vi "Strain Measurement.vi"(0 "Function":T5=enum."Update Sequence Status", 1 "Stress Sequence Parameters":T6={"Max Motor Position"=1380.0, "# Intermediate Points"=5000, "Initial Direction"=enum."Tension"} caption="Stress Parameters" {"# Intermediate Points" max=1390}, 2 "Which Program?":T1, 5 "Notifiers":T9, 7 "Message Queues":T22, 9 "Refnums":T7, 11 "error in (no error)":errorcluster, 12 "Track":bool) -> (6 "Sequence Progress":cluster{i32[], "Y":dbl[]}[](graph)=[{[0, 1, 2], "Y"=[-3.816391647148976e-15, -49.99999999999999, 0.0]}, {[3], "Y"=[50.0]}, {[4], "Y"=[-3.816391647148976e-15]}] caption="Strain Measurement Status", 15 "error out":errorcluster)   [LabVIEW 2014]
uses:
  support/Message Queue/All Message Queues.ctl
  support/Message Queue/Message Cluster.ctl
  support/Notifiers/Notifiers.ctl
  support/Message Handler Loop Notifiers.ctl
  Hardware Control/Parameter Analyzer/Parameter Analyzer Notifiers.ctl
  Hardware Control/Switching Matrix/Switching Matrix Notifiers.ctl
  Hardware Control/Stress Control/StressControl Notifiers.ctl
  Hardware Control/Spectrometer/Spectrometer Notifiers.ctl
  Hardware Control/Switches and Mirrors/SwitchesMirrors Notifiers.ctl
  Hardware Control/Camera/Camera Notifiers.ctl
  Hardware Control/XYZ Stage/XYZ Notifications.ctl
  Hardware Control/Autofocus/Autofocus Notifiers.ctl
  Optoelectronic Measurement/Optoelectronic Notifiers.ctl
  Save Data/SaveData Notifiers.ctl
  Instrument Sequence/Instrument Sequence Notifiers.ctl
  Strain Measurement Refnums.ctl
  Instrument Sequence/Action.ctl
  Instrument Sequence/Instrument List.ctl
  Plot Data/Electrical Data Plot Refnums.ctl
  Strain Measurement Function.ctl
  Instrument Sequence/Instrument Steps.ctl
  Instrument Sequence/Instrument Stequence - Which Program.ctl
  Hardware Control/Autofocus/AutoFocus Data.ctl
  Hardware Control/Autofocus/AutoFocus Config.ctl
  Hardware Control/Autofocus/ZScan.ctl
  <vilib>/Analysis/Matrix/Datatypes/RealMatrix.ctl
  Hardware Control/Autofocus/AutoFocus Refnums.ctl
  Hardware Control/Autofocus/Target Refnums.ctl
  Hardware Control/Autofocus/AutoFocus Initialize.ctl
  Hardware Control/Switches and Mirrors/SwitchesMirrors Config.ctl
  Hardware Control/Switches and Mirrors/SwitchesMirrors Status.ctl
  support/Message Queue/Message Queue.lvlib
  <vilib>/Analysis/Matrix/NI_Matrix.lvlib
panel:
  in  "Strain Measurement - Pause":bool
  out "Device ID":string caption="Instrument Sequence - Device ID"
  out "Device Information":string
  out "Instrument Steps":T2
  # "LICENSED MATERIALS – PROPERTY OF IBM\nCopyright IBM Corp. 2016,\nALL RIGHTS RESERVED"
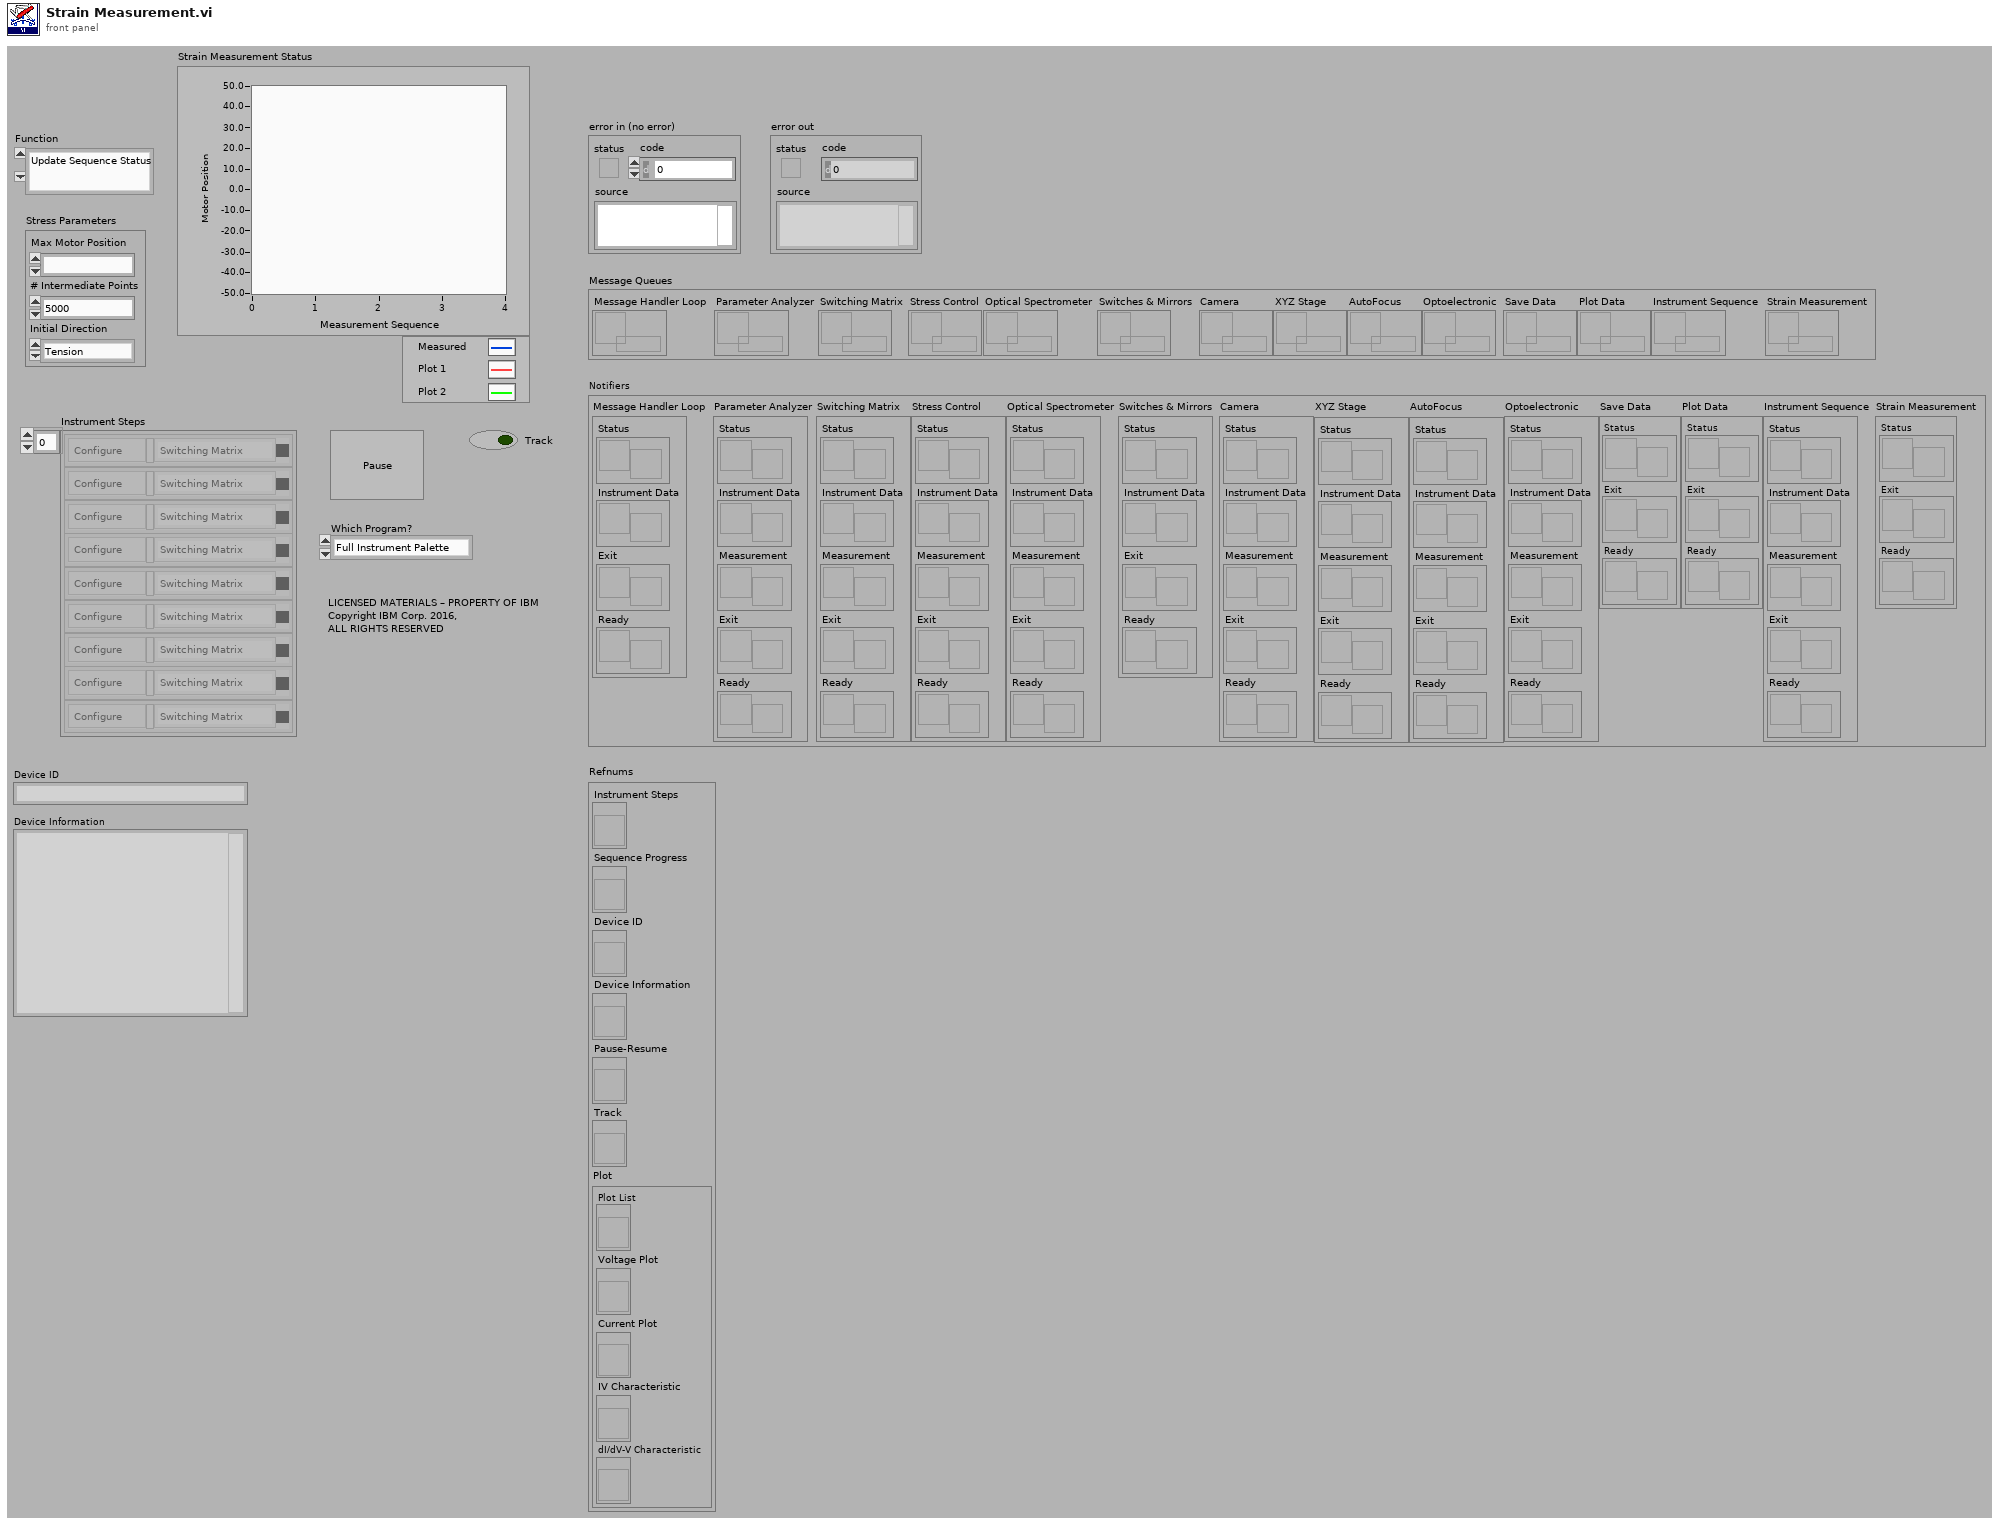
[diagram p1: front panel]
types:
  T1 = typedef "Instrument Stequence - Which Program.ctl" = enum16{"Full Instrument Palette", "Strain Electrical"}
  T2 = typedef "Instrument Steps.ctl" = cluster{"Action":T3, "Configuration":variant, "Instrument":T4, "Status":enum8{"False", "True", "Mixed"}}[]
  T3 = typedef "Action.ctl" = enum32{"Configure", "Measure"}
  T4 = typedef "Instrument List.ctl" = enum32{"Unknown Instrument", "Switching Matrix", "Parameter Analyzer", "Optical Spectrometer", "Optoelectronic", "Autofocus"}
  T5 = typedef "Strain Measurement Function.ctl" = enum16{"Get Stress Controller Status", "Define Strain Sequence", "Update Track", "Decide on Track", "Reset Strain Sequence", "Start Strain Measurement", "Set Strain Sequence Step", "Add Instrument Sequence Step", "Delete Instrument Sequence Step", "Clear Instrument Sequence", "Reset Instrument Sequence", "Load Instrument Sequence", "Save Instrument Sequence", "Measure Instrument Sequence", "Choose What Next", "Configure Stress Control", "Set Workspace Data", "Save to Workspace", "Update Sequence Status", "Pause", "Stop", "Update Refnums"}
  T6 = cluster{"Max Motor Position":ext, "# Intermediate Points":u32, "Initial Direction":enum16{"Tension", "Compression"}}
  T7 = typedef "Strain Measurement Refnums.ctl" = cluster{"Instrument Steps":refnum<vi>, "Sequence Progress":refnum<vi>, "Device ID":refnum<vi>, "Device Information":refnum<vi>, "Pause-Resume":refnum<vi>, "Track":refnum<vi>, "Plot":T8}
  T8 = typedef "Electrical Data Plot Refnums.ctl" = cluster{"Plot List":refnum<vi>, "Voltage Plot":refnum<vi>, "Current Plot":refnum<vi>, "IV Characteristic":refnum<vi>, "dI/dV-V Characteristic":refnum<vi>}
  T9 = typedef "Notifiers.ctl" = cluster{"Message Handler Loop":T10, "Parameter Analyzer":T11, "Switching Matrix":T12, "Stress Control":T13, "Optical Spectrometer":T14, "Switches & Mirrors":T15, "Camera":T16, "XYZ Stage":T17, "AutoFocus":T18, "Optoelectronic":T19, "Save Data":T20, "Plot Data":T20, "Instrument Sequence":T21, "Strain Measurement":cluster{"Status":refnum<notifier>, "Exit":refnum<notifier>, "Ready":refnum<notifier>}}
  T10 = typedef "Message Handler Loop Notifiers.ctl" = cluster{"Status":refnum<notifier>, "Instrument Data":refnum<notifier>, "Exit":refnum<notifier>, "Ready":refnum<notifier>}
  T11 = typedef "Parameter Analyzer Notifiers.ctl" = cluster{"Status":refnum<notifier>, "Instrument Data":refnum<notifier>, "Measurement":refnum<notifier>, "Exit":refnum<notifier>, "Ready":refnum<notifier>}
  T12 = typedef "Switching Matrix Notifiers.ctl" = cluster{"Status":refnum<notifier>, "Instrument Data":refnum<notifier>, "Measurement":refnum<notifier>, "Exit":refnum<notifier>, "Ready":refnum<notifier>}
  T13 = typedef "StressControl Notifiers.ctl" = cluster{"Status":refnum<notifier>, "Instrument Data":refnum<notifier>, "Measurement":refnum<notifier>, "Exit":refnum<notifier>, "Ready":refnum<notifier>}
  T14 = typedef "Spectrometer Notifiers.ctl" = cluster{"Status":refnum<notifier>, "Instrument Data":refnum<notifier>, "Measurement":refnum<notifier>, "Exit":refnum<notifier>, "Ready":refnum<notifier>}
  T15 = typedef "SwitchesMirrors Notifiers.ctl" = cluster{"Status":refnum<notifier>, "Instrument Data":refnum<notifier>, "Exit":refnum<notifier>, "Ready":refnum<notifier>}
  T16 = typedef "Camera Notifiers.ctl" = cluster{"Status":refnum<notifier>, "Instrument Data":refnum<notifier>, "Measurement":refnum<notifier>, "Exit":refnum<notifier>, "Ready":refnum<notifier>}
  T17 = typedef "XYZ Notifications.ctl" = cluster{"Status":refnum<notifier>, "Instrument Data":refnum<notifier>, "Measurement":refnum<notifier>, "Exit":refnum<notifier>, "Ready":refnum<notifier>}
  T18 = typedef "Autofocus Notifiers.ctl" = cluster{"Status":refnum<notifier>, "Instrument Data":refnum<notifier>, "Measurement":refnum<notifier>, "Exit":refnum<notifier>, "Ready":refnum<notifier>}
  T19 = typedef "Optoelectronic Notifiers.ctl" = cluster{"Status":refnum<notifier>, "Instrument Data":refnum<notifier>, "Measurement":refnum<notifier>, "Exit":refnum<notifier>, "Ready":refnum<notifier>}
  T20 = typedef "SaveData Notifiers.ctl" = cluster{"Status":refnum<notifier>, "Exit":refnum<notifier>, "Ready":refnum<notifier>}
  T21 = typedef "Instrument Sequence Notifiers.ctl" = cluster{"Status":refnum<notifier>, "Instrument Data":refnum<notifier>, "Measurement":refnum<notifier>, "Exit":refnum<notifier>, "Ready":refnum<notifier>}
  T22 = typedef "Message Queue.lvlib/All Message Queues.ctl" = cluster{"Message Handler Loop":refnum<queue>, "Parameter Analyzer":refnum<queue>, "Switching Matrix":refnum<queue>, "Stress Control":refnum<queue>, "Optical Spectrometer":refnum<queue>, "Switches & Mirrors":refnum<queue>, "Camera":refnum<queue>, "XYZ Stage":refnum<queue>, "AutoFocus":refnum<queue>, "Optoelectronic":refnum<queue>, "Save Data":refnum<queue>, "Plot Data":refnum<queue>, "Instrument Sequence":refnum<queue>, "Strain Measurement":refnum<queue>}
  T23 = cluster{"Wanna Track?":bool, "Makes Sense?":bool}
  T24 = typedef "AutoFocus Data.ctl" = cluster{"Configuration":T25, "Refnums":T28, "Initialize":T30}
  T25 = typedef "AutoFocus Config.ctl" = cluster{"Matching Criteria":cluster{"Minimum Score":sgl, "Color Score Weight":sgl, "Minimum Contrast":i32, "Match Mode":u32, "Match Feature Mode":u32, "Subpixel Accuracy":bool, "Color Sensitivity":u32, "Search Strategy":u32}, "Z Scan Parameters":T26, "Displacement":dbl, "Transformation Matrix":T27}
  T26 = typedef "ZScan.ctl" = cluster{"Z Range":ext, "Resolution":dbl, "Initial Direction":enum16{"Up", "Down"}, "Focus Threshold":dbl, "Ascent Constant":dbl}
  T27 = typedef "NI_Matrix.lvlib/RealMatrix.ctl" = dbl[][]
  T28 = typedef "AutoFocus Refnums.ctl" = cluster{"Instrument Status":refnum<vi>, "Matching Criteria":refnum<vi>, "Z Scan Parameters":refnum<vi>, "Distance":refnum<vi>, "Transformation Matrix":refnum<vi>, "Match and Edge":T29, "Matching Curves":refnum<vi>, "Tracking":refnum<vi>, "Focus":refnum<vi>, "Find Focus":refnum<vi>, "Set Target":refnum<vi>, "Link Stage & Camera":refnum<vi>, "Align":refnum<vi>}
  T29 = typedef "Target Refnums.ctl" = cluster{"Image":refnum<vi>, "Target":refnum<vi>, "Edge":refnum<vi>, "Target Data":refnum<vi>}
  T30 = typedef "AutoFocus Initialize.ctl" = cluster{"Update Refnums":bool, "Allocate Image Memory":bool, "Set Match Criteria":bool, "Link Stage & Camera":bool, "Set Target":bool, "Find Target":bool}
  T31 = enum8{"Enabled", "Disabled", "Disabled and Grayed Out"}
  T32 = typedef "SwitchesMirrors Config.ctl" = cluster{"Relay VISA Session":refnum<visa-resource-name>, "Switches":T33, "Delays (ms)":cluster{"Laser":u32, "Video":u32}}
  T33 = typedef "SwitchesMirrors Status.ctl" = cluster{"Laser":bool, "Video":bool}
  T34 = typedef "StressControl Config.ctl" = cluster{"Stress Control VISA Session":refnum<visa-resource-name>, "Axis":i32, "Motion":u16, "Destination (°)":dbl, "Speed (°/s)":dbl, "Position (°)":dbl}
  T35 = typedef "SaveData Workspace Info.ctl" = cluster{"Device Name":string, "Device Info":string, "Path":path}
  T36 = typedef "StressControl Data.ctl" = cluster{"Configuration":T34, "Refnums":T37, "Initialization":T38}
  T37 = typedef "StressControl Refnums.ctl" = cluster{"Instrument Status":refnum<vi>, "Position":refnum<vi>, "Mecahnism Motion":refnum<vi>, "Destination":refnum<vi>, "Apply Stress":refnum<vi>, "Stop":refnum<vi>, "Stress Control VISA":refnum<vi>}
  T38 = typedef "StressControl Initialization.ctl" = cluster{"Update Visa Session":bool, "Update Configuration":bool, "Update Refnums":bool, "Get Position":bool}
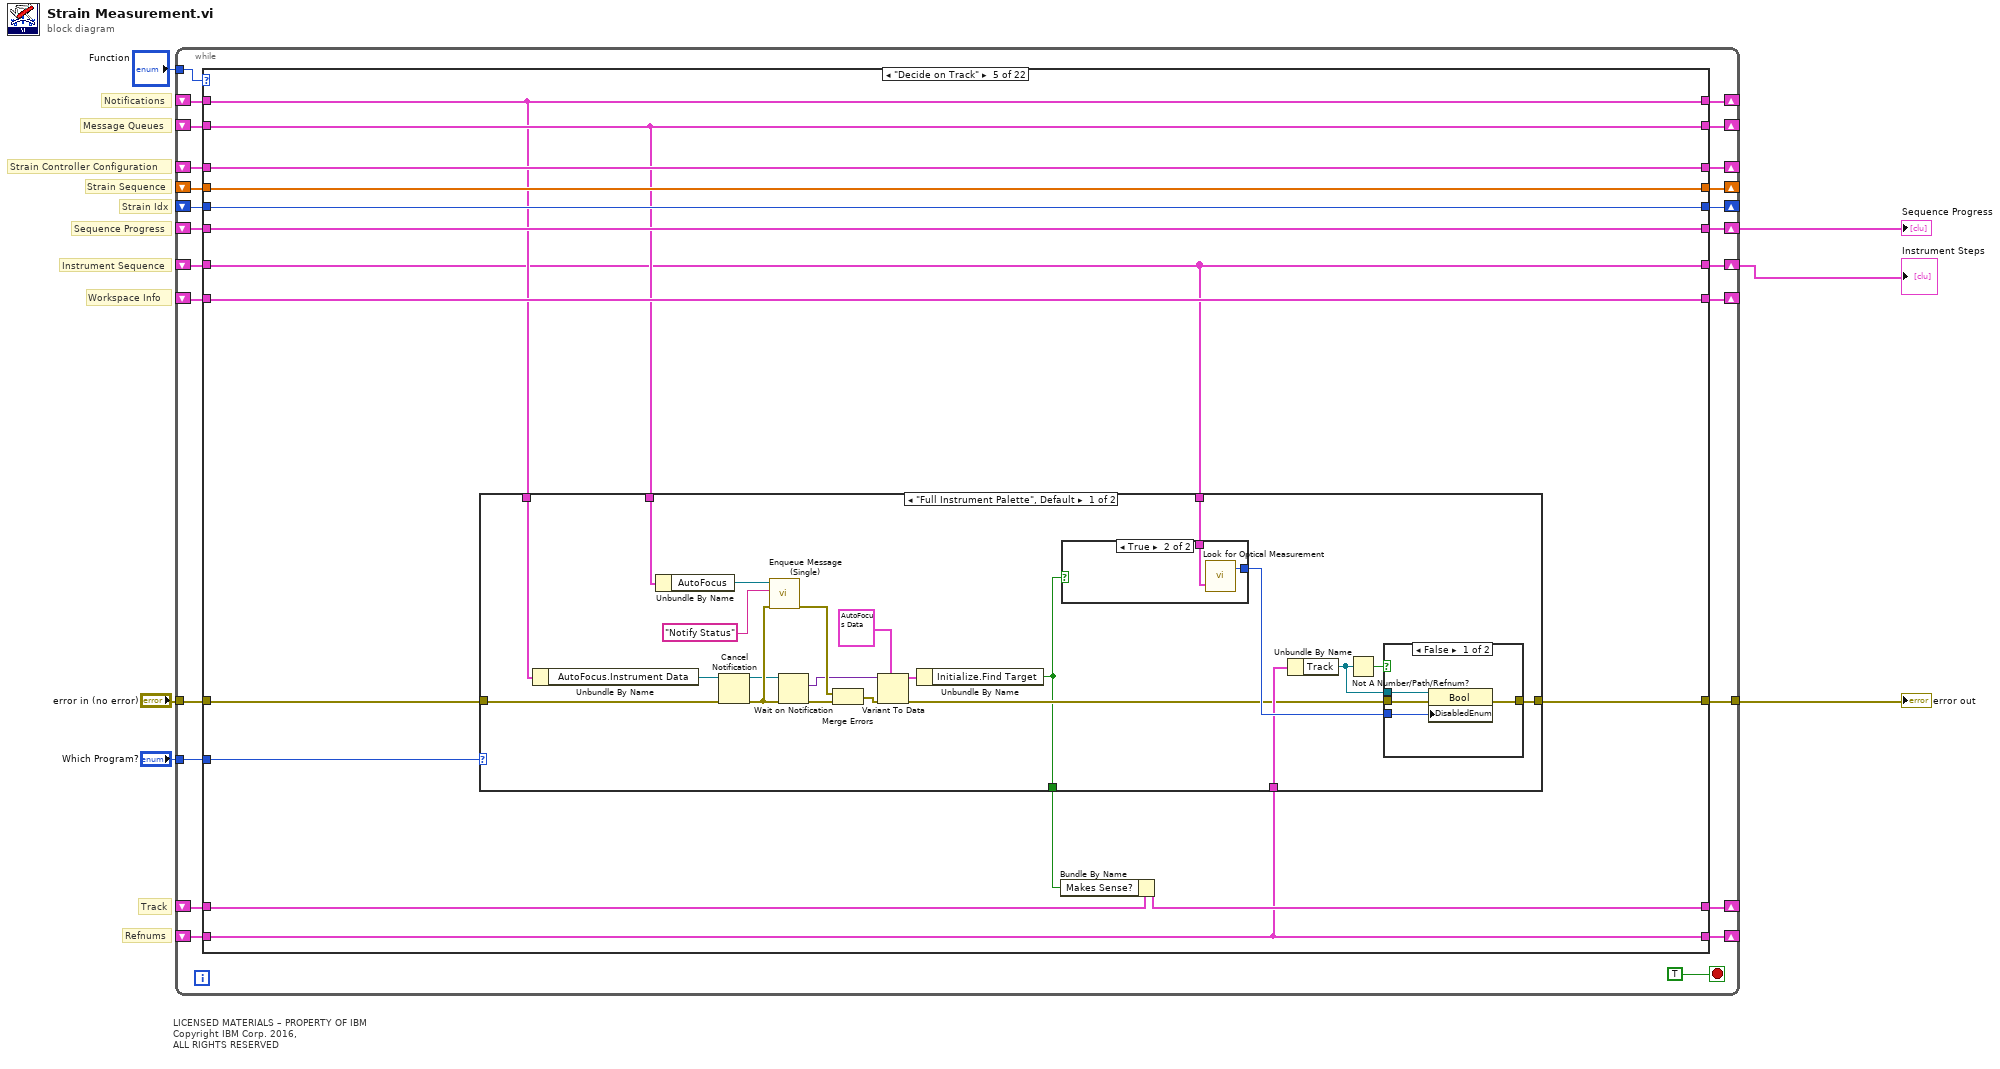
[diagram p0: block diagram]
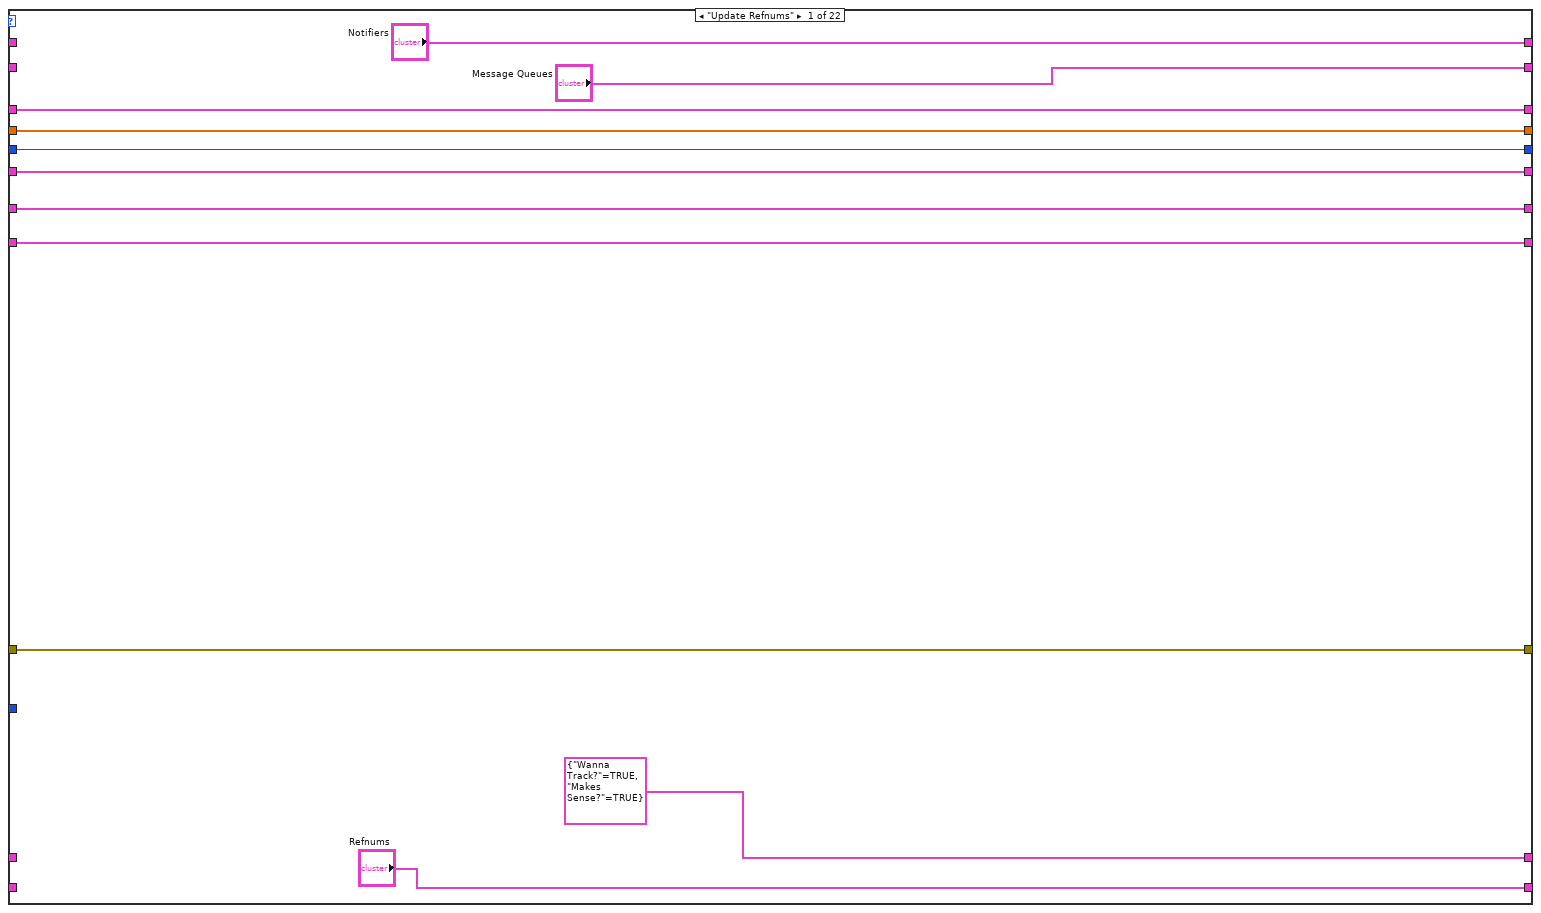
[diagram p2: hidden frame]
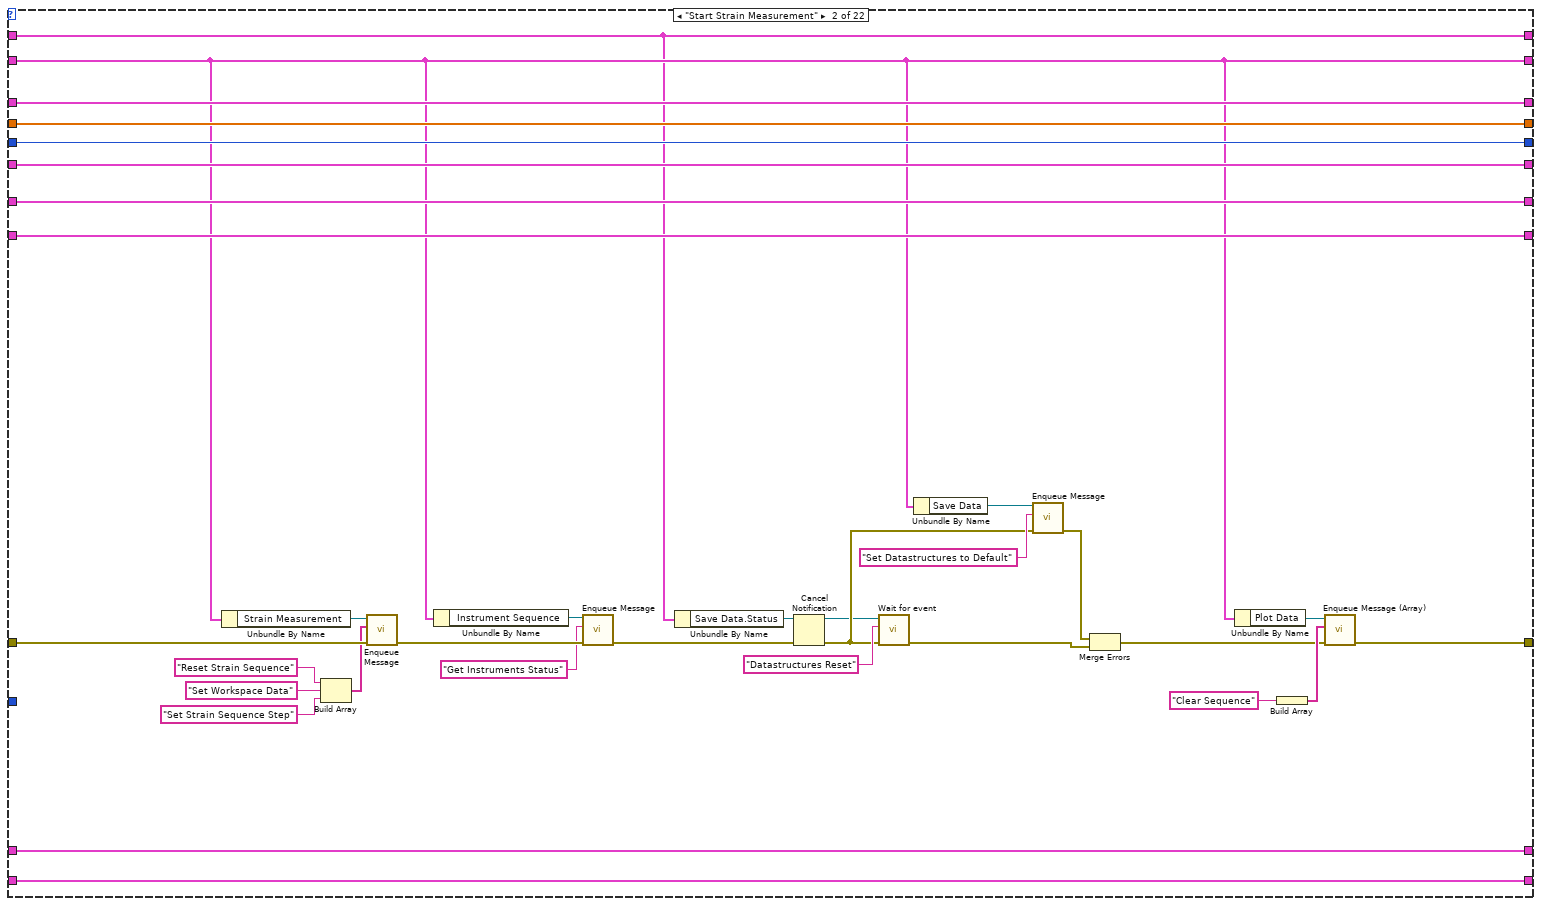
[diagram p3: hidden frame]
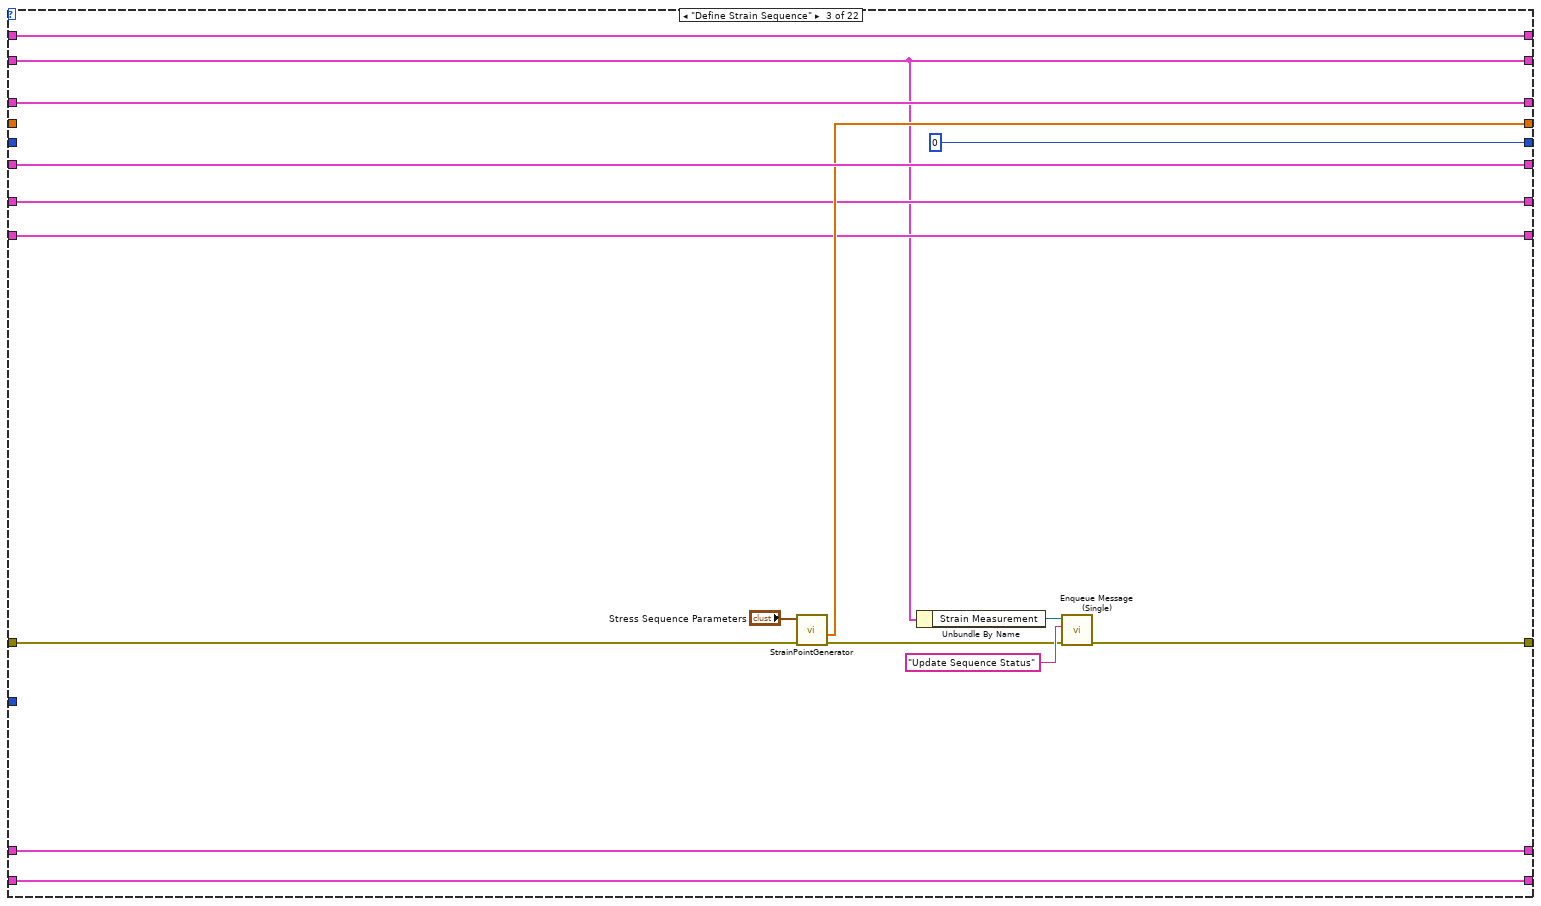
[diagram p4: hidden frame]
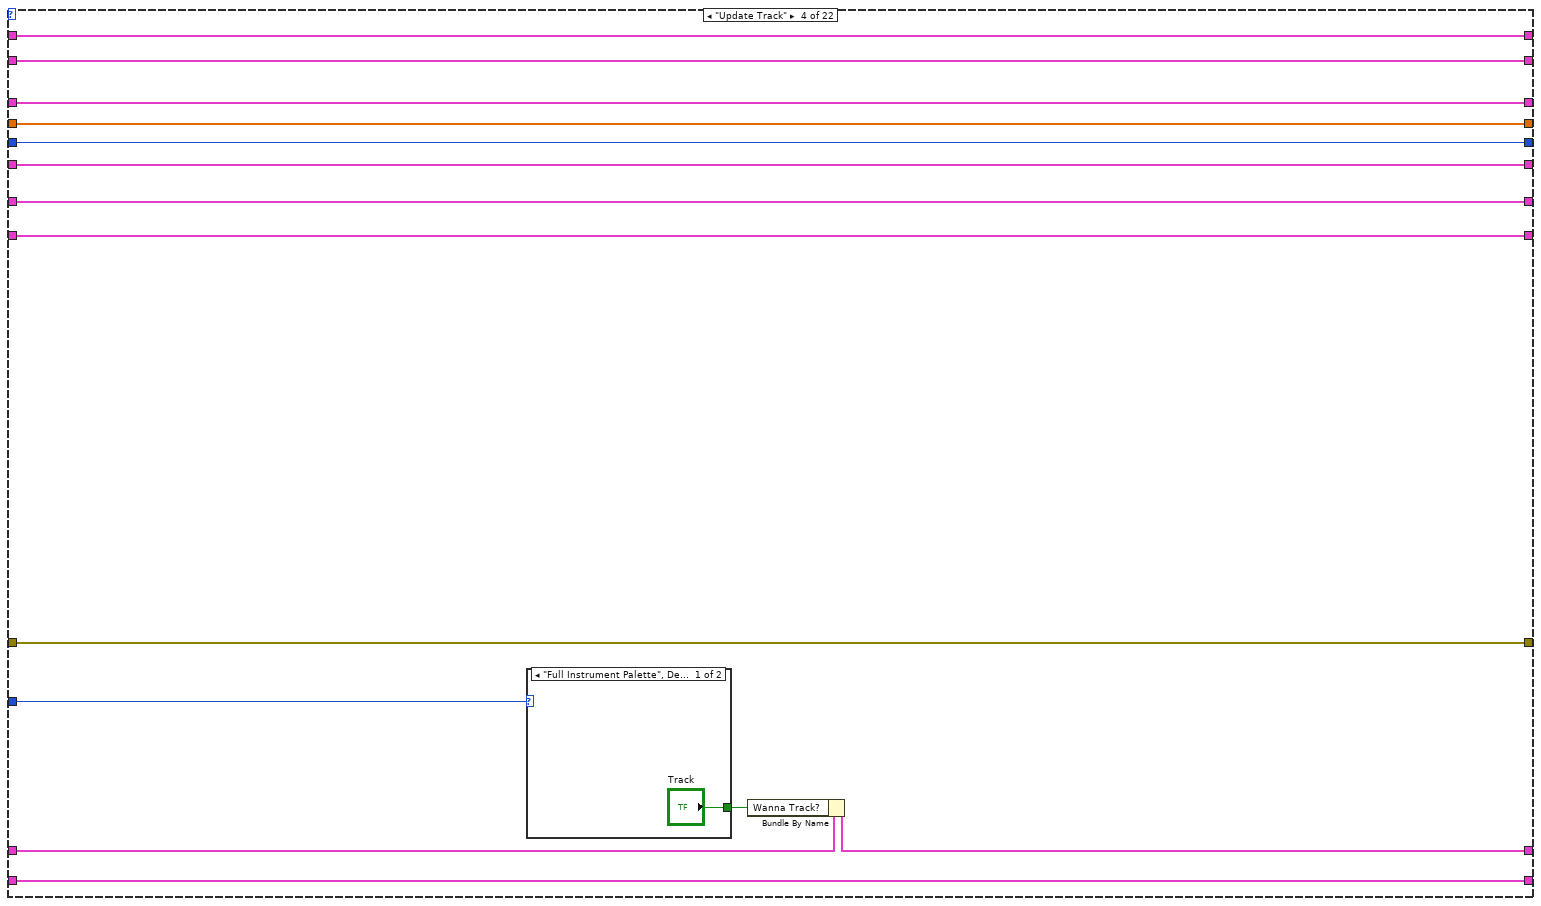
[diagram p5: hidden frame]
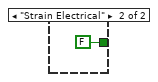
[diagram p6: hidden frame]
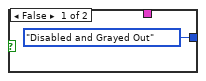
[diagram p7: hidden frame]
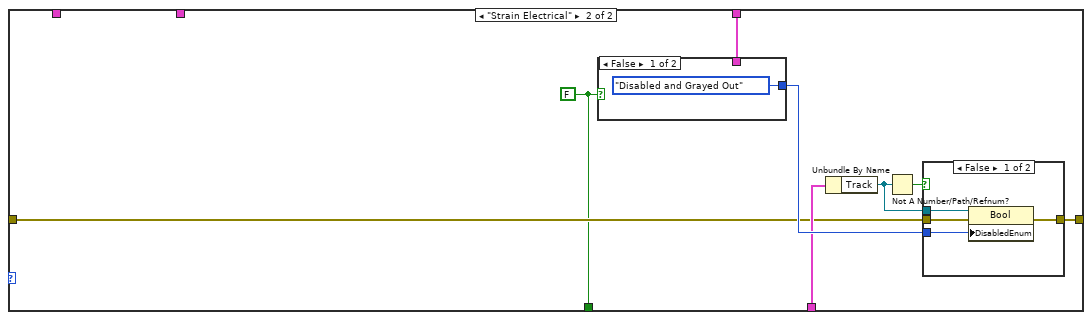
[diagram p9: hidden frame]
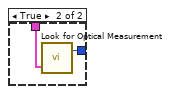
[diagram p10: hidden frame]
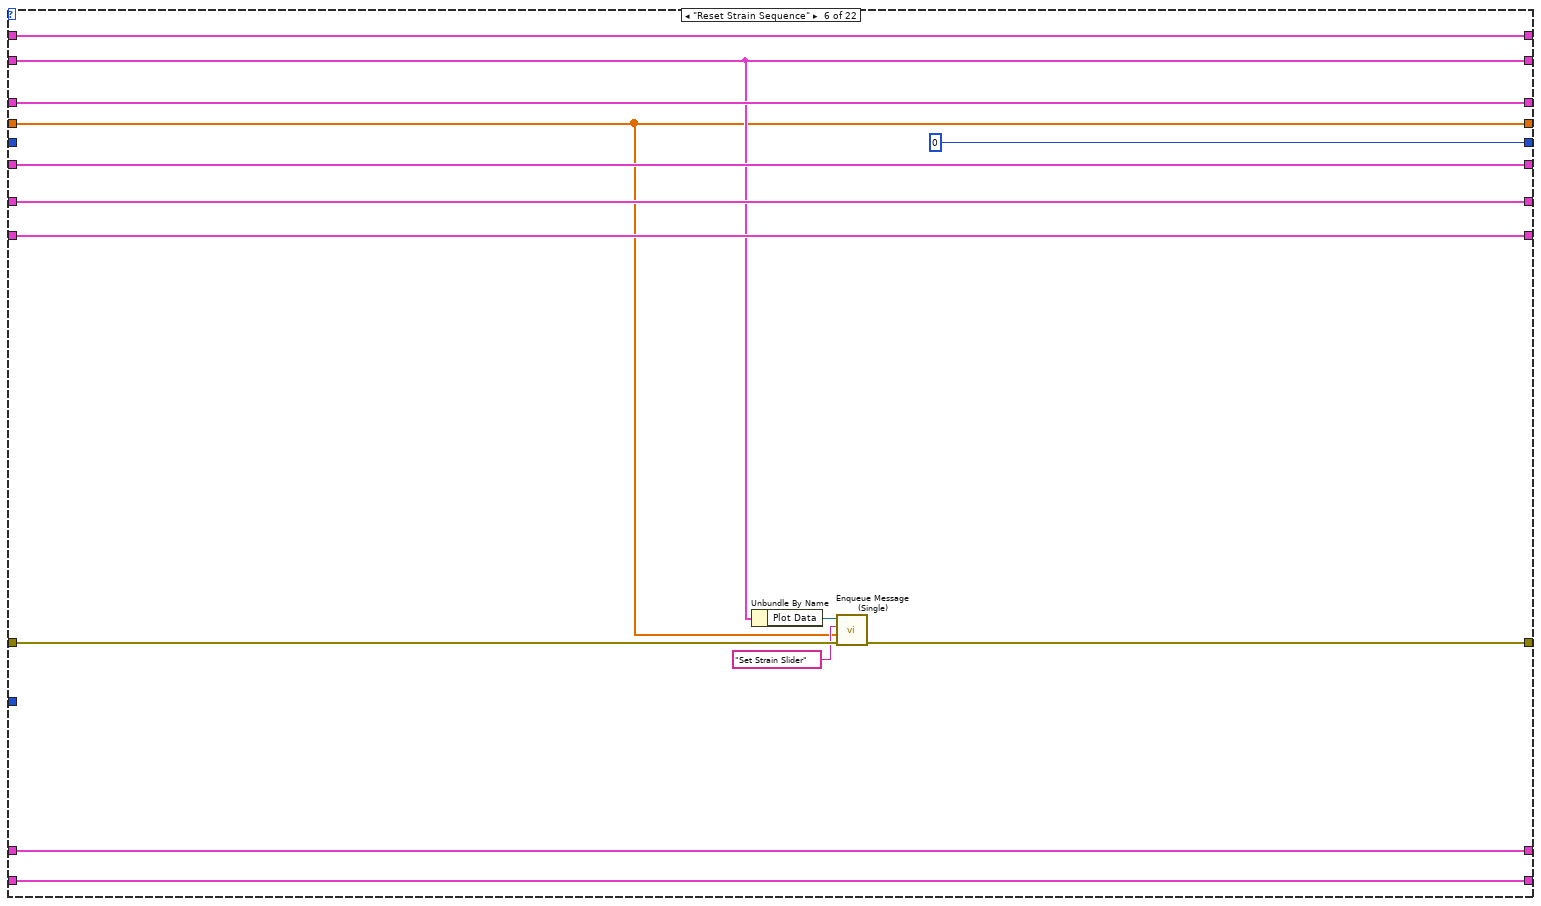
[diagram p12: hidden frame]
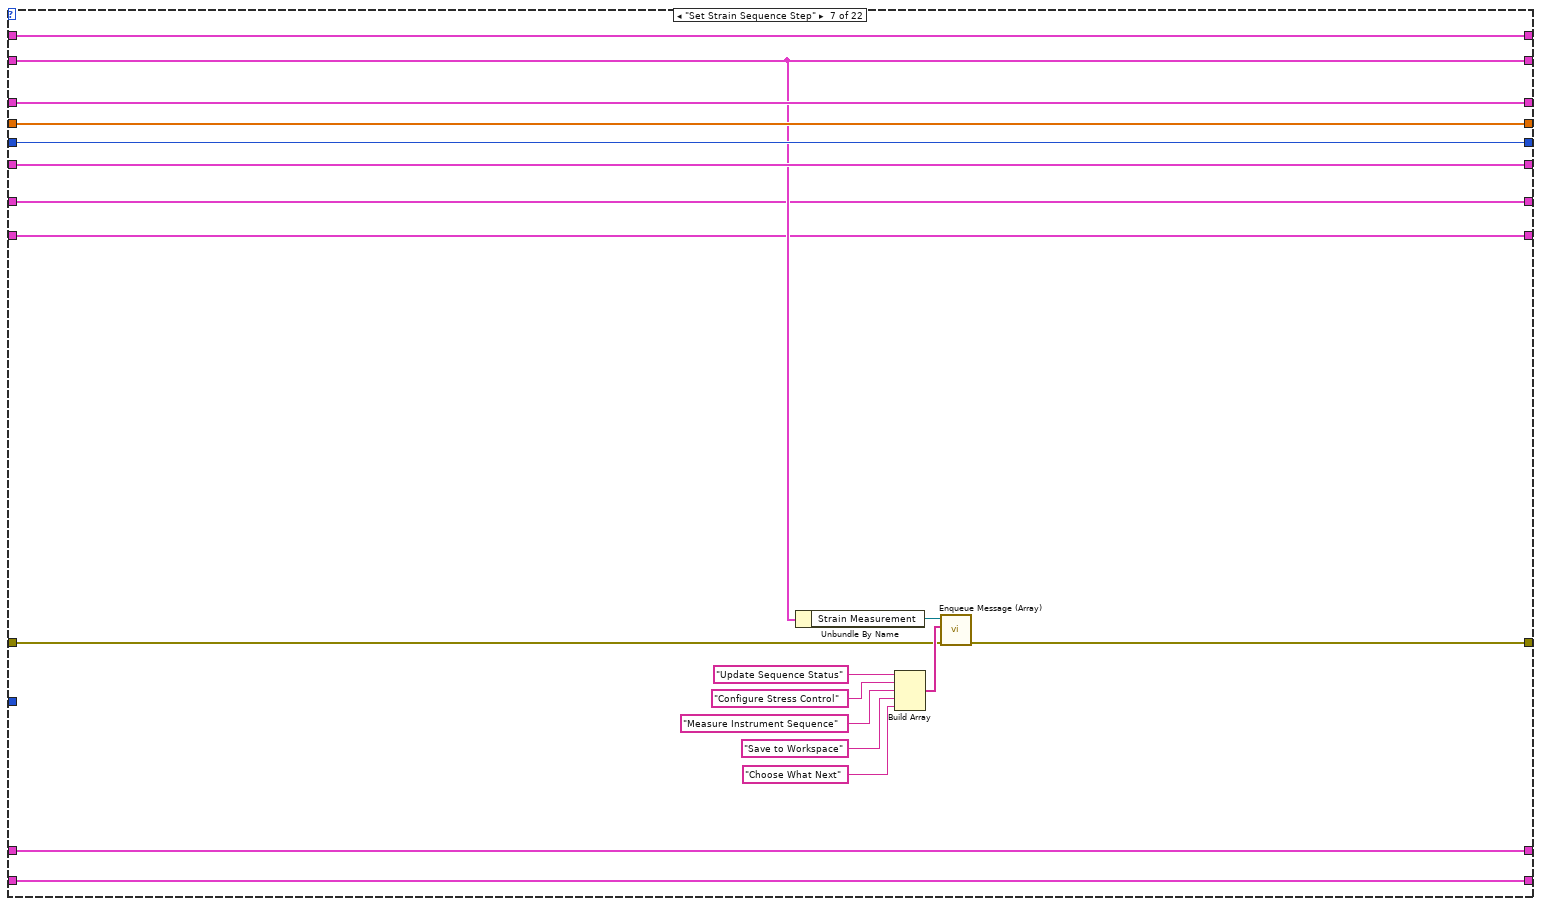
[diagram p13: hidden frame]
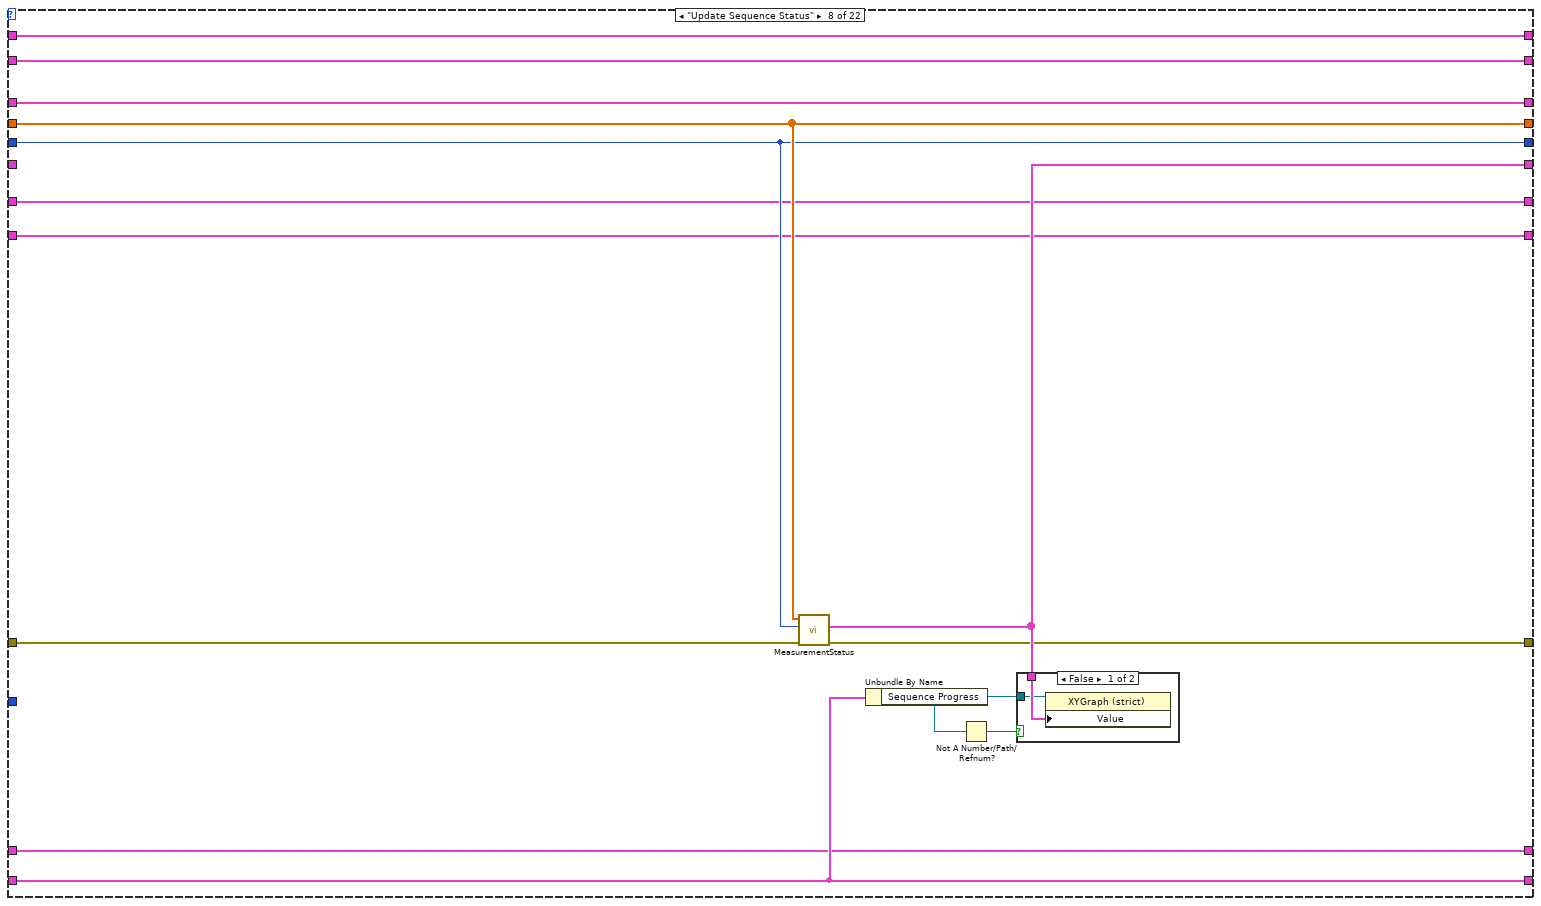
[diagram p14: hidden frame]
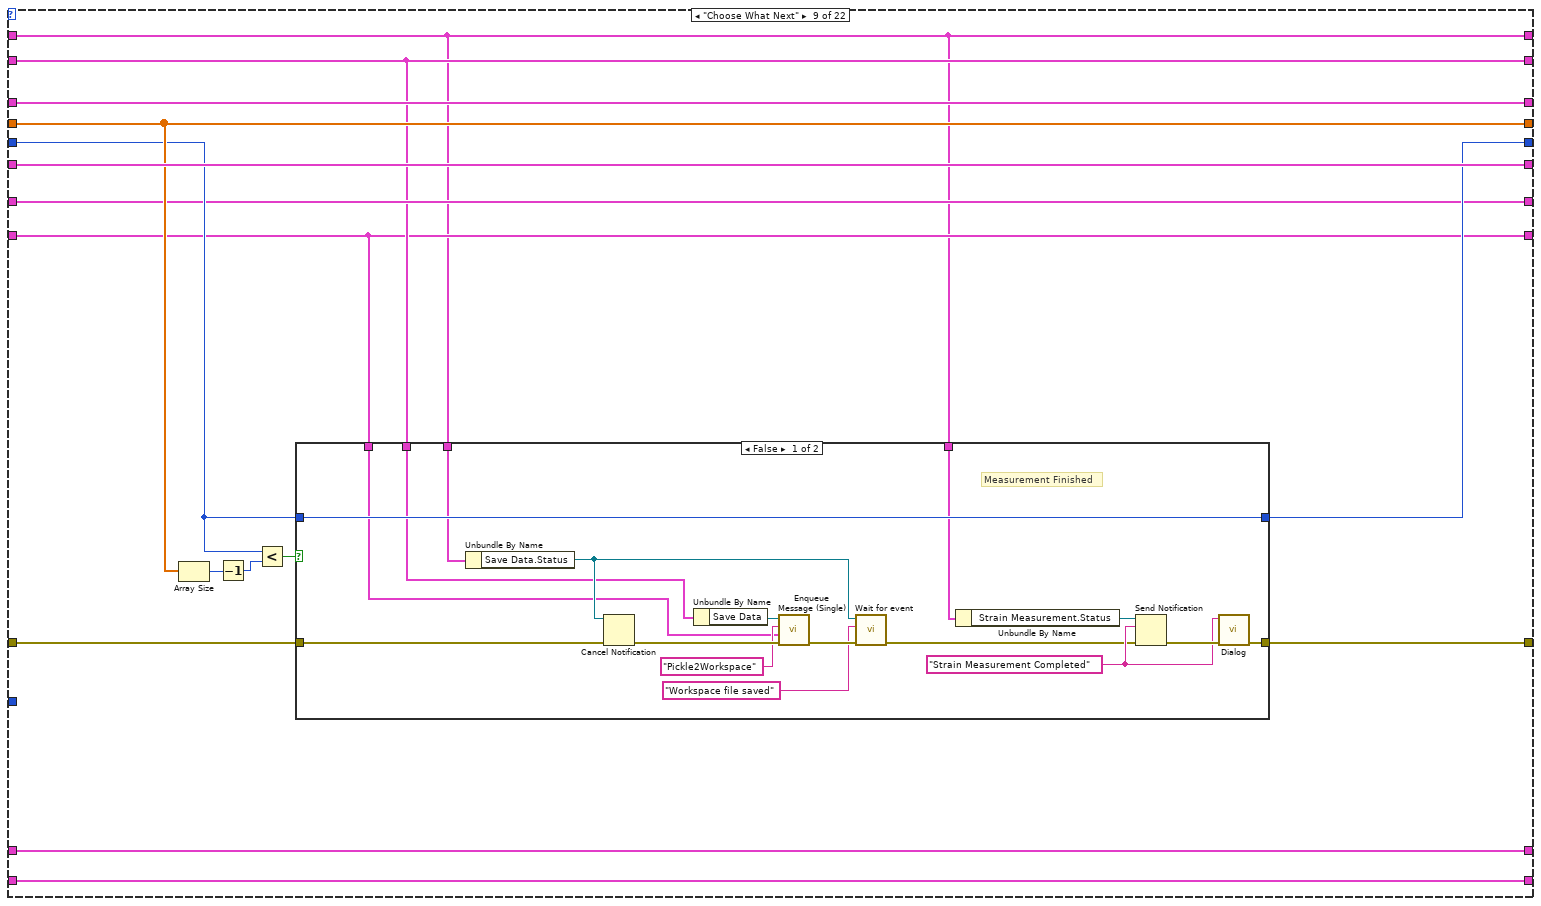
[diagram p16: hidden frame]
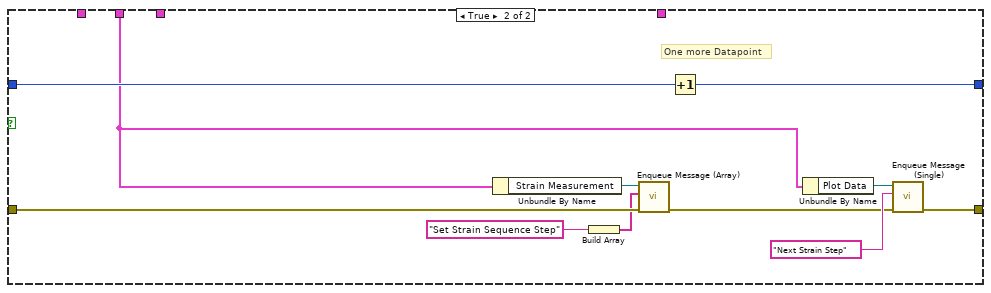
[diagram p17: hidden frame]
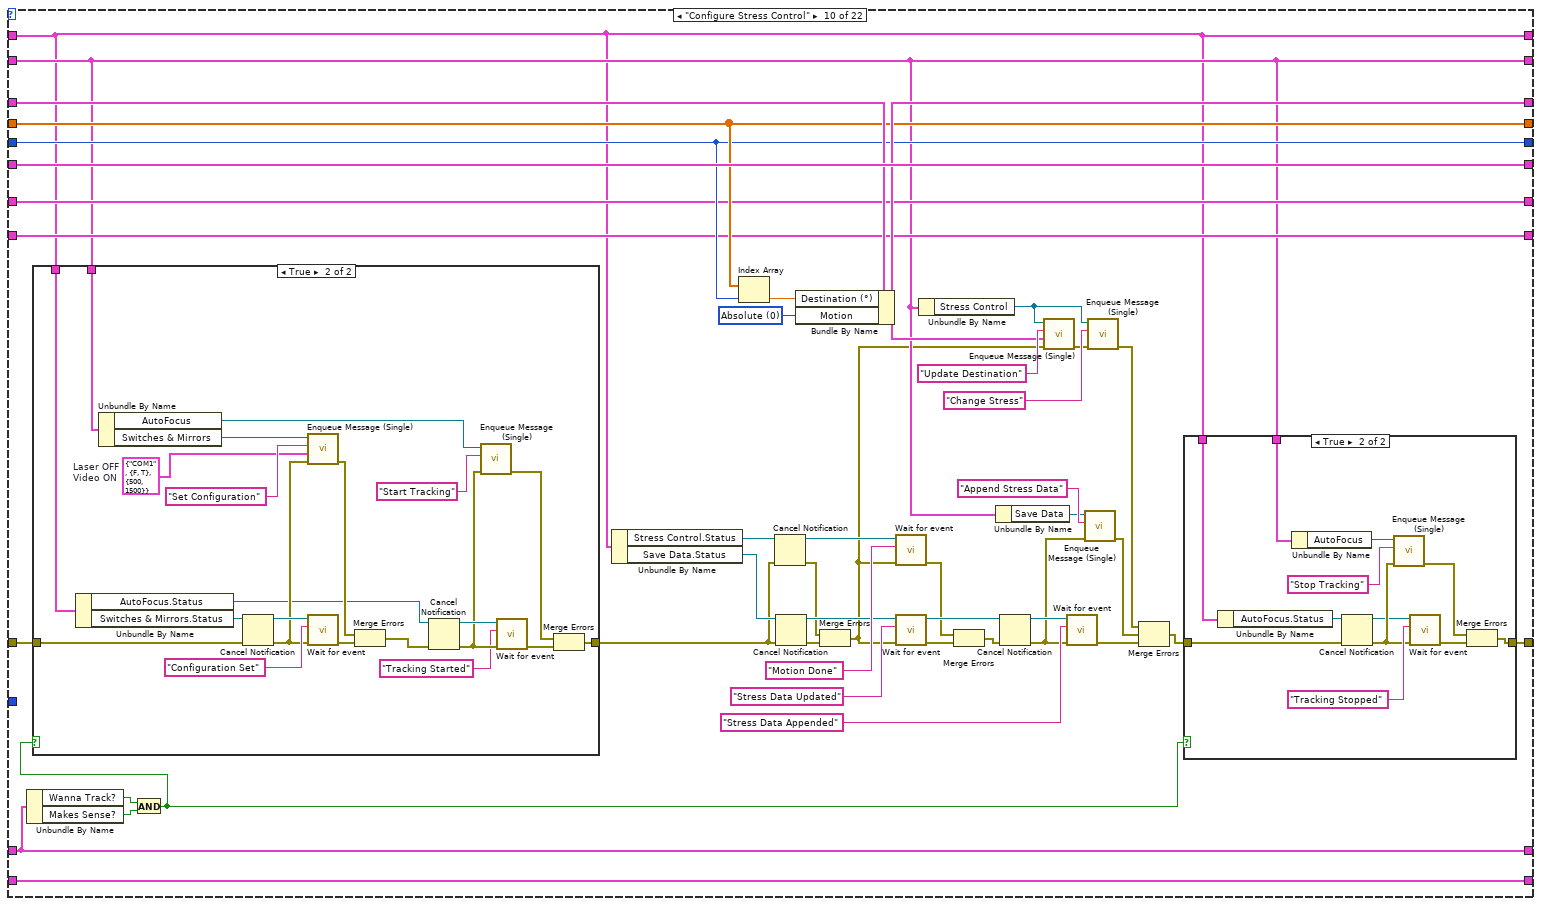
[diagram p18: hidden frame]
diagram:
  # "LICENSED MATERIALS – PROPERTY OF IBM\nCopyright IBM Corp. 2016,\nALL RIGHTS RESERVED"
  # "Track"
  # "Instrument Sequence"
  # "Workspace Info"
  # "Refnums"
  # "Strain Controller Configuration"
  # "Message Queues"
  # "Notifications"
  # "Strain Sequence"
  # "Sequence Progress"
  # "Strain Idx"
  n1 = while {
    tunnel: "error in (no error)" -> [w31]
    tunnel: [w30] -> w5
    tunnel: "Function" -> [w29]
    shift-right: [w24] -> _
    shift-left: _ -> [w25]
    shift-right: [w23] -> _
    shift-left: _ -> [w28]
    shift-right: [w22] -> _
    shift-left: _ -> [w27]
    shift-right: [w21] -> w4
    shift-left: _ -> [w20]
    shift-right: [w18] -> _
    shift-left: _ -> [w19]
    shift-right: [w17] -> _
    shift-left: _ -> [w16]
    shift-right: [w15] -> _
    shift-left: _ -> [w14]
    shift-right: [w12] -> _
    shift-left: _ -> [w13]
    shift-right: [w11] -> w3
    shift-left: _ -> [w10]
    shift-right: [w8] -> _
    shift-left: _ -> [w9]
    tunnel: "Which Program?" -> [w7]
    stop <- TRUE stop-if-true
    n2 = case shown="\"Decide on Track\"" w29 {
      tunnel: w31 -> [w42 w68 w91 w98 w114 w173 w188 w215 w228 w290 w356 w415 w450 w477 w504 w534 w564 w594 w622 w647 w660 w671]
      tunnel: [w42 w60 w77 w98 w110 w169 w194 w205 w231 w288 w348 w416 w448 w482 w487 w517 w547 w577 w611 w636 w661 w668] -> w30
      tunnel: w28 -> [_ w50 w89 w104 w113 w181 w200 w211 w218 w284 w349 w412 w451 w480 w502 w532 w562 w592 w619 w646 w667 w680]
      tunnel: w27 -> [_ w52 w80 w99 w115 w175 w187 w210 w221 w287 w360 w403 w456 w479 w505 w535 w565 w595 w623 w648 w662 w670]
      tunnel: [w36 w73 w84 w102 w121 w178 w191 w208 w225 w297 w372 w411 w464 w465 w511 w541 w571 w601 w629 w654 w666 w679] -> w15
      tunnel: ["Refnums" w75 w90 w105 w111 w182 w201 w213 w230 w300 w364 w406 w460 w481 w494 w524 w554 w584 w610 w644 w659 w675] -> w24
      tunnel: w25 -> [_ w75 w90 w105 w111 w182 w201 w213 w230 w300 w364 w406 w460 w481 w494 w524 w554 w584 w610 w644 w659 w675]
      tunnel: ["Notifiers" w50 w89 w104 w113 w181 w200 w211 w218 w284 w349 w412 w451 w480 w502 w532 w562 w592 w619 w646 w667 w680] -> w23
      tunnel: ["Message Queues" w52 w80 w99 w115 w175 w187 w210 w221 w287 w360 w403 w456 w479 w505 w535 w565 w595 w623 w648 w662 w670] -> w22
      tunnel: [w41 w74 w88 w103 w122 w180 w199 w209 w229 w299 w369 w408 w461 w478 w508 w538 w568 w598 w626 w651 w663 w676] -> w21
      tunnel: w20 -> [w41 w74 w88 w103 w122 w180 w199 _ w229 w299 w369 w408 w461 w478 w508 w538 w568 w598 w626 w651 w663 w676]
      tunnel: w19 -> [w40 w72 _ w97 w119 w171 w190 w207 w226 w296 w371 w410 w463 w476 w510 w540 w570 w600 w628 w653 w665 w678]
      tunnel: [w40 w72 w86 w97 w119 w171 w190 w207 w226 w296 w371 w410 w463 w476 w510 w540 w570 w600 w628 w653 w665 w678] -> w18
      tunnel: [w35 w71 0 ("Numer of Points") w96 w118 0 ("Numer of Points") w189 w206 w223 w295 w370 w409 w462 w471 w509 w539 w569 w599 w627 w652 w664 w677] -> w17
      tunnel: w16 -> [w35 w71 _ w96 w118 _ w189 w206 w224 w295 w370 w409 w462 w471 w509 w539 w569 w599 w627 w652 w664 w677]
      tunnel: w14 -> [w36 w73 w84 w102 w121 w178 w191 w208 w225 w298 w372 w411 w464 _ w511 w541 w571 w601 w629 w654 w666 w679]
      tunnel: w13 -> [w34 w70 w83 w101 w120 w177 w185 w204 w220 w294 w368 _ w457 w470 w496 w526 w556 w586 w609 w643 w657 w674]
      tunnel: [w34 w70 w83 w101 w120 w177 w185 w204 w220 w294 w368 w407 w457 w470 w496 w526 w556 w586 w609 w643 w657 w674] -> w12
      tunnel: [w33 w65 w82 w100 w112 w176 w184 w203 w222 w291 w362 w405 w455 w469 w493 w523 w553 w583 w607 w642 w656 w673] -> w11
      tunnel: w10 -> [w33 w65 w82 w100 w112 w176 w184 w203 w222 w291 w362 w405 w455 w469 _ _ _ _ _ w642 w656 w673]
      tunnel: w9 -> [_ w59 w76 w95 w117 w170 w183 w202 w219 w283 w351 w404 w454 w468 w495 w525 w555 w585 w608 w641 w655 w669]
      tunnel: [T23 {"Wanna Track?"=TRUE, "Makes Sense?"=TRUE} w59 w76 w94 w116 w170 w183 w202 w219 w283 w351 w404 w454 w468 w495 w525 w555 w585 w608 w641 w655 w669] -> w8
      tunnel: w7 -> [_ _ _ w92 w108 _ _ _ _ _ _ _ _ _ _ _ _ _ _ _ _ _]
      frame "Update Refnums" {
      }
      frame "Start Strain Measurement" {
        n3 = Unbundle By Name(w52) -> ("Strain Measurement"=w69:refnum<queue>)
        n4 = Build Array("Reset Strain Sequence" ("Message"), "Set Workspace Data" ("Message"), "Set Strain Sequence Step" ("Message")) -> (w57:string[])
        n5 = call-poly "Enqueue Message.vi"("error in (no error)"=w68, "Message Array"=w57, "Message Queue"=w69) -> ("error out"=w58:errorcluster)  [unwired: 7 in, 1 out]
        n6 = Unbundle By Name(w52) -> ("Instrument Sequence"=w56:refnum<queue>)
        n7 = call-poly "Enqueue Message.vi"("error in (no error)"=w58, "Message"="Get Instruments Status", "Message Queue"=w56) -> ("error out"=w47:errorcluster)  [unwired: 7 in, 1 out]
        n8 = Unbundle By Name(w50) -> ("Save Data.Status"=w51:refnum<notifier>)
        n9 = Cancel Notification(0:w51, 3:w47) -> (8:w43:refnum<notifier>, 11:w45:errorcluster)  [unwired: 1 out]
        n10 = call "Wait for event.vi"("error in (no error)"=w45, "String"="Datastructures Reset", "Notifier in"=w43) -> ("error out"=w44:errorcluster)  [unwired: 7 in, 1 out]
        n11 = Unbundle By Name(w52) -> ("Save Data"=w53:refnum<queue>)
        n12 = call-poly "Enqueue Message.vi"("error in (no error)"=w45, "Message"="Set Datastructures to Default", "Message Queue"=w53) -> ("error out"=w49:errorcluster)  [unwired: 7 in, 1 out]
        n13 = Merge Errors(w49, w44) -> (w48:errorcluster)
        n14 = Unbundle By Name(w52) -> ("Plot Data"=w61:refnum<queue>)
        n15 = Build Array("Clear Sequence" ("Message")) -> (w62:string[])
        n16 = call "Enqueue Message (Array).vi"("error in (no error)"=w48, "Message Array"=w62, "Message Queue"=w61) -> ("error out"=w60:errorcluster)  [unwired: 1 in, 7 out]
      }
      frame "Define Strain Sequence" {
        n17 = call "StrainPointGenerator.vi"("error in (no error)"=w91, "Strain Sweep Parameters"="Stress Sequence Parameters") -> ("error out"=w78:errorcluster, "Strain Points"=w86:dbl[])  [unwired: 8 out]
        n18 = Unbundle By Name(w80) -> ("Strain Measurement"=w81:refnum<queue>)
        n19 = call "Enqueue Message (Single).vi"("error in (no error)"=w78, "Message"="Update Sequence Status", "Message Queue"=w81) -> ("error out"=w77:errorcluster)  [unwired: 1 in, 7 out]
      }
      frame "Update Track" {
        n20 = case shown="\"Full Instrument Palette\", Default" w92 {
          tunnel: ["Track" FALSE ("Track")] -> w93
          frame "Full Instrument Palette", Default {
          }
          frame "Strain Electrical" {
          }
        }
        n21 = Bundle By Name(cluster=w95, "Wanna Track?"=w93) -> (w94:T23)
      }
      frame "Decide on Track" {
        n22 = case shown="\"Full Instrument Palette\", Default" w108 {
          tunnel: w115 -> [w144 _]
          tunnel: w114 -> [w143 w154]
          tunnel: w113 -> [w142 _]
          tunnel: w112 -> [w127 w157]
          tunnel: w111 -> [w126 w156]
          tunnel: [w124 w155] -> w110
          tunnel: [w123 w153] -> w109
          frame "Full Instrument Palette", Default {
            n23 = Unbundle By Name(w142) -> ("AutoFocus.Instrument Data"=w139:refnum<notifier>)
            n24 = Unbundle By Name(w144) -> ("AutoFocus"=w140:refnum<queue>)
            n25 = Cancel Notification(0:w139, 3:w143) -> (8:w134:refnum<notifier>, 11:w135:errorcluster)  [unwired: 1 out]
            n26 = call "Enqueue Message (Single).vi"("error in (no error)"=w135, "Message"="Notify Status", "Message Queue"=w140) -> ("error out"=w137:errorcluster)  [unwired: 1 in, 7 out]
            n27 = Wait on Notification(notifier=w134, error in (no error)=w135) -> (notification=w133:variant, error out=w136:errorcluster)  [unwired: 2 in, 2 out]
            n28 = Merge Errors(w137, w136) -> (w138:errorcluster)
            n29 = Variant To Data(error in=w138, type=T24 {"Configuration"={"Matching Criteria"={"Minimum Score"=700.0, "Color Score Weight"=700.0, "Minimum Contrast"=50, "Match Mode"=0, "Match Feature Mode"=0, "Subpixel Accuracy"=TRUE, "Color Sensitivity"=1, "Search Strategy"=1}, "Z Scan Parameters"={"Z Range"=1380.0, "Resolution"=5000.0, "Initial Direction"=enum."Up", "Focus Threshold"=0.1, "Ascent Constant"=0.1}, "Displacement"=0.0, "Transformation Matrix"=[]}, "Refnums"={"Instrument Status"=refnum, "Matching Criteria"=refnum, "Z Scan Parameters"=refnum, "Distance"=refnum, "Transformation Matrix"=refnum, "Match and Edge"={"Image"=refnum, "Target"=refnum, "Edge"=refnum, "Target Data"=refnum}, "Matching Curves"=refnum, "Tracking"=refnum, "Focus"=refnum, "Find Focus"=refnum, "Set Target"=refnum, "Link Stage & Camera"=refnum, "Align"=refnum}, "Initialize"={"Update Refnums"=FALSE, "Allocate Image Memory"=FALSE, "Set Match Criteria"=FALSE, "Link Stage & Camera"=FALSE, "Set Target"=FALSE, "Find Target"=FALSE}} ("AutoFocus Data"), Variant=w133) -> (data=w131:T24, error out=w125:errorcluster)
            n30 = Unbundle By Name(w131) -> ("Initialize.Find Target"=w123:bool)
            n31 = case shown="True" w123 {
              tunnel: [T31."Disabled and Grayed Out" ("Enabled") w147] -> w128
              tunnel: w127 -> [_ w146]
              frame False {
              }
              frame True {
                n32 = call "Look for Optical Measurement.vi"("Instrument Steps in"=w146) -> ("Enabled"=w147:T31)  [unwired: 1 in, 1 out]
              }
            }
            n33 = Unbundle By Name(w126) -> ("Track"=w129:refnum<vi>)
            n34 = Not A Number/Path/Refnum?(number/path/refnum=w129) -> (NaN/Path/Refnum?=w130:bool)
            n35 = case shown="False" w130 {
              tunnel: w129 -> [w151 _]
              tunnel: [w150 w152] -> w124
              tunnel: w128 -> [w149 _]
              tunnel: w125 -> [w148 w152]
              frame False {
                n36 = property class="Bool"(reference=w151, error in=w148, "DisabledEnum"=w149) -> (error out=w150:errorcluster)  [unwired: 1 out]
              }
              frame True {
              }
            }
          }
          frame "Strain Electrical" {
            w153 = FALSE
            n37 = case shown="False" w153 {
              tunnel: [T31."Disabled and Grayed Out" ("Enabled") w163] -> w158
              tunnel: w157 -> [_ w162]
              frame False {
              }
              frame True {
                n38 = call "Look for Optical Measurement.vi"("Instrument Steps in"=w162) -> ("Enabled"=w163:T31)  [unwired: 1 in, 1 out]
              }
            }
            n39 = Unbundle By Name(w156) -> ("Track"=w159:refnum<vi>)
            n40 = Not A Number/Path/Refnum?(number/path/refnum=w159) -> (NaN/Path/Refnum?=w160:bool)
            n41 = case shown="False" w160 {
              tunnel: w159 -> [w167 _]
              tunnel: [w166 w168] -> w155
              tunnel: w158 -> [w165 _]
              tunnel: w154 -> [w164 w168]
              frame False {
                n42 = property class="Bool"(reference=w167, error in=w164, "DisabledEnum"=w165) -> (error out=w166:errorcluster)  [unwired: 1 out]
              }
              frame True {
              }
            }
          }
        }
        n43 = Bundle By Name(cluster=w117, "Makes Sense?"=w109) -> (w116:T23)
      }
      frame "Reset Strain Sequence" {
        n44 = Unbundle By Name(w175) -> ("Plot Data"=w174:refnum<queue>)
        n45 = call "Enqueue Message (Single).vi"("error in (no error)"=w173, "Message Data"=w171, "Message"="Set Strain Slider", "Message Queue"=w174) -> ("error out"=w169:errorcluster)  [unwired: 7 out]
      }
      frame "Set Strain Sequence Step" {
        n46 = Unbundle By Name(w187) -> ("Strain Measurement"=w186:refnum<queue>)
        n47 = Build Array("Update Sequence Status" ("Message"), "Configure Stress Control" ("Message"), "Measure Instrument Sequence" ("Message"), "Save to Workspace" ("Message"), "Choose What Next" ("Message")) -> (w195:string[])
        n48 = call "Enqueue Message (Array).vi"("error in (no error)"=w188, "Message Array"=w195, "Message Queue"=w186) -> ("error out"=w194:errorcluster)  [unwired: 1 in, 7 out]
      }
      frame "Update Sequence Status" {
        n49 = call "MeasurementStatus.vi"("error in (no error)"=w215, "Current Measurement Idx"=w206, "Measurement Sequence"=w207) -> ("error out"=w205:errorcluster, "Sequence Progress"=w209:cluster{i32[], "Y":dbl[]}[])  [unwired: 7 out]
        n50 = Unbundle By Name(w213) -> ("Sequence Progress"=w214:refnum<vi>)
        n51 = Not A Number/Path/Refnum?(number/path/refnum=w214) -> (NaN/Path/Refnum?=w212:bool)
        n52 = case shown="False" w212 {
          tunnel: w209 -> [w217 _]
          tunnel: w214 -> [w216 _]
          frame False {
            n53 = property on="Property Node" class="XYGraph (strict)"(reference=w216, "Value"=w217) -> ()  [unwired: 1 in, 2 out]
          }
          frame True {
          }
        }
      }
      frame "Choose What Next" {
        n54 = Array Size(array=w226) -> (size(s)=w227:i32)
        n55 = Decrement(x=w227) -> (x-1=w233:i32)
        n56 = Less?(x=w224, y=w233) -> (x < y?=w232:bool)
        n57 = case shown="False" w232 {
          tunnel: w228 -> [w238 w259]
          tunnel: [w247 w252] -> w231
          tunnel: [w250 w261] -> w223
          tunnel: w224 -> [w250 w260]
          tunnel: w218 -> [w249 _]
          tunnel: w221 -> [w235 w253]
          tunnel: w220 -> [w234 _]
          tunnel: w218 -> [w236 _]
          frame False {
            w245 = "Strain Measurement Completed" ("message")
            # "Measurement Finished"
            n58 = Unbundle By Name(w236) -> ("Save Data.Status"=w243:refnum<notifier>)
            n59 = Cancel Notification(0:w243, 3:w238) -> (11:w241:errorcluster)  [unwired: 2 out]
            n60 = Unbundle By Name(w235) -> ("Save Data"=w239:refnum<queue>)
            n61 = call "Enqueue Message (Single).vi"("error in (no error)"=w241, "Message Data"=w234, "Message"="Pickle2Workspace", "Message Queue"=w239) -> ("error out"=w244:errorcluster)  [unwired: 7 out]
            n62 = call "Wait for event.vi"("error in (no error)"=w244, "String"="Workspace file saved", "Notifier in"=w243) -> ("error out"=w237:errorcluster)  [unwired: 7 in, 1 out]
            n63 = Unbundle By Name(w249) -> ("Strain Measurement.Status"=w248:refnum<notifier>)
            n64 = Send Notification(notification=w245, notifier=w248, error in (no error)=w237) -> (error out=w246:errorcluster)  [unwired: 1 out]
            n65 = call "Dialog.vi"("error in (no error)"=w246, "message"=w245) -> ("error out"=w247:errorcluster)  [unwired: 1 in, 8 out]
          }
          frame True {
            # "One more Datapoint"
            n66 = Unbundle By Name(w253) -> ("Strain Measurement"=w258:refnum<queue>)
            n67 = Build Array("Set Strain Sequence Step" ("Message")) -> (w256:string[])
            n68 = call "Enqueue Message (Array).vi"("error in (no error)"=w259, "Message Array"=w256, "Message Queue"=w258) -> ("error out"=w251:errorcluster)  [unwired: 1 in, 7 out]
            n69 = Increment(x=w260) -> (x+1=w261:i32)
            n70 = Unbundle By Name(w253) -> ("Plot Data"=w254:refnum<queue>)
            n71 = call "Enqueue Message (Single).vi"("error in (no error)"=w251, "Message"="Next Strain Step", "Message Queue"=w254) -> ("error out"=w252:errorcluster)  [unwired: 2 in, 6 out]
          }
        }
      }
      frame "Configure Stress Control" {
        w301 = u16 0 items=["Absolute", "Relative"] ("Mechanism Motion")
        n72 = Unbundle By Name(w283) -> ("Wanna Track?"=w282:bool, "Makes Sense?"=w281:bool)
        n73 = And(x=w282, y=w281) -> (x .and. y?=w280:bool)
        n74 = case shown="True" w280 {
          tunnel: w287 -> [_ w329]
          tunnel: [w320 w325] -> w276
          tunnel: w290 -> [w320 w324]
          tunnel: w284 -> [_ w328]
          frame False {
          }
          frame True {
            w326 = T32 {"Relay VISA Session"="COM1", "Switches"={"Laser"=FALSE, "Video"=TRUE}, "Delays (ms)"={"Laser"=500, "Video"=1500}}  # Laser OFF Video ON
            n75 = Unbundle By Name(w328) -> ("AutoFocus.Status"=w321:refnum<notifier>, "Switches & Mirrors.Status"=w339:refnum<notifier>)
            n76 = Unbundle By Name(w329) -> ("AutoFocus"=w322:refnum<queue>, "Switches & Mirrors"=w341:refnum<queue>)
            n77 = Cancel Notification(0:w339, 3:w324) -> (8:w338:refnum<notifier>, 11:w336:errorcluster)  [unwired: 1 out]
            n78 = call "Enqueue Message (Single).vi"("error in (no error)"=w336, "Message Data"=w326, "Message"="Set Configuration", "Message Queue"=w341) -> ("error out"=w335:errorcluster)  [unwired: 7 out]
            n79 = call "Wait for event.vi"("error in (no error)"=w336, "String"="Configuration Set", "Notifier in"=w338) -> ("error out"=w337:errorcluster)  [unwired: 7 in, 1 out]
            n80 = Merge Errors(w335, w337) -> (w323:errorcluster)
            n81 = Cancel Notification(0:w321, 3:w323) -> (8:w334:refnum<notifier>, 11:w332:errorcluster)  [unwired: 1 out]
            n82 = call "Enqueue Message (Single).vi"("error in (no error)"=w332, "Message"="Start Tracking", "Message Queue"=w322) -> ("error out"=w333:errorcluster)  [unwired: 1 in, 7 out]
            n83 = call "Wait for event.vi"("error in (no error)"=w332, "String"="Tracking Started", "Notifier in"=w334) -> ("error out"=w331:errorcluster)  [unwired: 7 in, 1 out]
            n84 = Merge Errors(w333, w331) -> (w325:errorcluster)
          }
        }
        n85 = Unbundle By Name(w284) -> ("Stress Control.Status"=w279:refnum<notifier>, "Save Data.Status"=w278:refnum<notifier>)
        n86 = Index Array(array=w296, index=w295) -> (element=w302:dbl)
        n87 = Cancel Notification(0:w279, 3:w276) -> (8:w277:refnum<notifier>, 11:w263:errorcluster)  [unwired: 1 out]
        n88 = Cancel Notification(0:w278, 3:w276) -> (8:w275:refnum<notifier>, 11:w274:errorcluster)  [unwired: 1 out]
        n89 = Bundle By Name(cluster=w298, "Destination (°)"=w302, "Motion"=w301) -> (w297:T34)
        n90 = Merge Errors(w263, w274) -> (w262:errorcluster)
        n91 = call "Wait for event.vi"("error in (no error)"=w262, "String"="Motion Done", "Notifier in"=w277) -> ("error out"=w265:errorcluster)  [unwired: 7 in, 1 out]
        n92 = call "Wait for event.vi"("error in (no error)"=w262, "String"="Stress Data Updated", "Notifier in"=w275) -> ("error out"=w267:errorcluster, "Notifier out"=w271:refnum<notifier>)  [unwired: 7 in]
        n93 = Unbundle By Name(w287) -> ("Stress Control"=w303:refnum<queue>)
        n94 = Merge Errors(w265, w267) -> (w266:errorcluster)
        n95 = Unbundle By Name(w287) -> ("Save Data"=w292:refnum<queue>)
        n96 = Cancel Notification(0:w271, 3:w266) -> (8:w270:refnum<notifier>, 11:w264:errorcluster)  [unwired: 1 out]
        n97 = call "Enqueue Message (Single).vi"("error in (no error)"=w262, "Message Data"=w297, "Message"="Update Destination", "Message Queue"=w303) -> ("error out"=w304:errorcluster)  [unwired: 7 out]
        n98 = call "Wait for event.vi"("error in (no error)"=w264, "String"="Stress Data Appended", "Notifier in"=w270) -> ("error out"=w268:errorcluster)  [unwired: 7 in, 1 out]
        n99 = call "Enqueue Message (Single).vi"("error in (no error)"=w264, "Message"="Append Stress Data", "Message Queue"=w292) -> ("error out"=w272:errorcluster)  [unwired: 1 in, 7 out]
        n100 = call "Enqueue Message (Single).vi"("error in (no error)"=w304, "Message"="Change Stress", "Message Queue"=w303) -> ("error out"=w286:errorcluster)  [unwired: 1 in, 7 out]
        n101 = Merge Errors(w286, w272, w268) -> (w289:errorcluster)
        n102 = case shown="True" w280 {
          tunnel: w287 -> [_ w319]
          tunnel: [w307 w311] -> w288
          tunnel: w289 -> [w307 w309]
          tunnel: w284 -> [_ w315]
          frame False {
          }
          frame True {
            n103 = Unbundle By Name(w315) -> ("AutoFocus.Status"=w314:refnum<notifier>)
            n104 = Unbundle By Name(w319) -> ("AutoFocus"=w318:refnum<queue>)
            n105 = Cancel Notification(0:w314, 3:w309) -> (8:w308:refnum<notifier>, 11:w312:errorcluster)  [unwired: 1 out]
            n106 = call "Enqueue Message (Single).vi"("error in (no error)"=w312, "Message"="Stop Tracking", "Message Queue"=w318) -> ("error out"=w310:errorcluster)  [unwired: 1 in, 7 out]
            n107 = call "Wait for event.vi"("error in (no error)"=w312, "String"="Tracking Stopped", "Notifier in"=w308) -> ("error out"=w313:errorcluster)  [unwired: 7 in, 1 out]
            n108 = Merge Errors(w310, w313) -> (w311:errorcluster)
          }
        }
      }
      frame "Measure Instrument Sequence" {
        n109 = Unbundle By Name(w349) -> ("Instrument Sequence.Instrument Data"=w352:refnum<notifier>, "Instrument Sequence.Status"=w353:refnum<notifier>)
        n110 = Cancel Notification(0:w352, 3:w356) -> (11:w354:errorcluster)  [unwired: 2 out]
        n111 = Cancel Notification(0:w353, 3:w356) -> (11:w355:errorcluster)  [unwired: 2 out]
        n112 = Merge Errors(w354, w355) -> (w357:errorcluster)
        n113 = while {
          tunnel: w353 -> [w382]
          tunnel: w352 -> [w381]
          tunnel: w364 -> [w376]
          shift-right: [w383] -> w365
          shift-left: w357 -> [w375]
          stop <- w373 stop-if-true
          n114 = Wait on Notification(notifier=w382, error in (no error)=w375) -> (notification=w378:variant, error out=w380:errorcluster)  [unwired: 4 out]
          n115 = Variant To Data(error in=w380, type="", Variant=w378) -> (data=w374:string, error out=w379:errorcluster)
          n116 = case shown="\"Instrument Sequence Completed\"" w374 {
            tunnel: [w384 w386 w401] -> w383
            tunnel: w381 -> [_ w393 _]
            tunnel: w379 -> [w384 w392 w401]
            tunnel: w376 -> [_ w387 _]
            tunnel: [_ _ TRUE] -> w373
            frame Default {
            }
            frame "Instrument Sequence Reset", "Instrument Sequence Updated" {
              n117 = Wait on Notification(notifier=w393, error in (no error)=w392) -> (notification=w394:variant, error out=w395:errorcluster)  [unwired: 4 out]
              n118 = Unbundle By Name(w387) -> ("Instrument Steps"=w389:refnum<vi>)
              n119 = Variant To Data(error in=w395, type=T2 [] ("Instrument Steps 2"), Variant=w394) -> (data=w388:T2, error out=w385:errorcluster)
              n120 = Not A Number/Path/Refnum?(number/path/refnum=w389) -> (NaN/Path/Refnum?=w390:bool)
              n121 = case shown="False" w390 {
                tunnel: w389 -> [w399 _]
                tunnel: w388 -> [w398 _]
                tunnel: [w397 w400] -> w386
                tunnel: w385 -> [w396 w400]
                frame False {
                  n122 = property class="Arr (strict)"(reference=w399, error in=w396, "Value"=w398) -> (error out=w397:errorcluster)  [unwired: 1 out]
                }
                frame True {
                }
              }
            }
            frame "Instrument Sequence Completed" {
            }
          }
        }
        n123 = Unbundle By Name(w360) -> ("Instrument Sequence"=w367:refnum<queue>)
        n124 = call "Enqueue Message (Single).vi"("error in (no error)"=w357, "Message"="Start Sequence for Strain Measurement", "Message Queue"=w367) -> ("error out"=w363:errorcluster)  [unwired: 1 in, 7 out]
        n125 = Unbundle By Name(w349) -> ("Save Data.Status"=w346:refnum<notifier>)
        n126 = Merge Errors(w363, w365) -> (w344:errorcluster)
        n127 = Cancel Notification(0:w346, 3:w344) -> (8:w345:refnum<notifier>, 11:w343:errorcluster)  [unwired: 1 out]
        n128 = Unbundle By Name(w360) -> ("Save Data"=w359:refnum<queue>)
        n129 = call "Wait for event.vi"("error in (no error)"=w343, "String"="Stress Measurement Step Appended", "Notifier in"=w345) -> ("error out"=w347:errorcluster)  [unwired: 7 in, 1 out]
        n130 = call "Enqueue Message (Single).vi"("error in (no error)"=w343, "Message"="Append Stress Measurement Step", "Message Queue"=w359) -> ("error out"=w361:errorcluster)  [unwired: 1 in, 7 out]
        n131 = Merge Errors(w361, w347) -> (w348:errorcluster)
      }
      frame "Set Workspace Data" {
        n132 = call "Set Device Information.vi"() -> ("error out"=w417:errorcluster, "Workspace Info"=w407:T35, "OK?"=w414:bool)  [unwired: 9 out]
        n133 = Merge Errors(w417, w415) -> (w413:errorcluster)
        n134 = case shown="True" w414 {
          tunnel: [w420 w429] -> w416
          tunnel: w407 -> [_ w428]
          tunnel: w413 -> [w421 w427]
          tunnel: w406 -> [_ w424]
          tunnel: w403 -> [w419 _]
          frame False {
            n135 = Unbundle By Name(w419) -> ("Strain Measurement"=w422:refnum<queue>)
            n136 = call "Enqueue Message (Single).vi"("Priority Message? (F)"=TRUE, "error in (no error)"=w421, "Message"="Stop", "Message Queue"=w422) -> ("error out"=w420:errorcluster)  [unwired: 1 in, 6 out]
          }
          frame True {
            n137 = Unbundle By Name(w424) -> ("Device ID"=w432:refnum<vi>, "Device Information"=w434:refnum<vi>)
            n138 = Unbundle By Name(w428) -> ("Device Name"=w426:string, "Device Info"=w425:string)
            "Device Information" <- w425
            "Device ID" <- w426
            n139 = Not A Number/Path/Refnum?(number/path/refnum=w432) -> (NaN/Path/Refnum?=w431:bool)
            n140 = case shown="False" w431 {
              tunnel: [w443 w444] -> w430
              tunnel: w426 -> [w442 _]
              tunnel: w432 -> [w441 _]
              tunnel: w427 -> [w440 w444]
              frame False {
                n141 = property class="Str"(reference=w441, error in=w440, "Value"=w442) -> (error out=w443:errorcluster)  [unwired: 1 out]
              }
              frame True {
              }
            }
            n142 = Not A Number/Path/Refnum?(number/path/refnum=w434) -> (NaN/Path/Refnum?=w433:bool)
            n143 = case shown="False" w433 {
              tunnel: w430 -> [w438 w439]
              tunnel: [w437 w439] -> w429
              tunnel: w425 -> [w436 _]
              tunnel: w434 -> [w435 _]
              frame False {
                n144 = property class="Str"(reference=w435, error in=w438, "Value"=w436) -> (error out=w437:errorcluster)  [unwired: 1 out]
              }
              frame True {
              }
            }
          }
        }
      }
      frame "Save to Workspace" {
        n145 = Unbundle By Name(w451) -> ("Save Data.Status"=w452:refnum<notifier>)
        n146 = Cancel Notification(0:w452, 3:w450) -> (8:w446:refnum<notifier>, 11:w447:errorcluster)  [unwired: 1 out]
        n147 = Unbundle By Name(w456) -> ("Save Data"=w458:refnum<queue>)
        n148 = call "Enqueue Message (Single).vi"("error in (no error)"=w447, "Message Data"=w457, "Message"="Save Stress Measurement", "Message Queue"=w458) -> ("error out"=w445:errorcluster)  [unwired: 7 out]
        n149 = call "Wait for event.vi"("error in (no error)"=w447, "String"="Stress Measurement Saved", "Notifier in"=w446) -> ("error out"=w449:errorcluster)  [unwired: 7 in, 1 out]
        n150 = Merge Errors(w445, w449) -> (w448:errorcluster)
      }
      frame "Get Stress Controller Status" {
        n151 = Unbundle By Name(w480) -> ("Stress Control.Instrument Data"=w472:refnum<notifier>)
        n152 = Cancel Notification(0:w472, 3:w477) -> (11:w473:errorcluster)  [unwired: 2 out]
        n153 = Wait on Notification(notifier=w472, error in (no error)=w473) -> (notification=w485:variant, error out=w486:errorcluster)  [unwired: 4 out]
        n154 = call "StressControl Data.vi"() -> ("Stress Control Data"=w467:T36)
        n155 = Variant To Data(error in=w486, type=w467, Variant=w485) -> (data=w466:T36, error out=w475:errorcluster)
        n156 = Unbundle By Name(w479) -> ("Stress Control"=w484:refnum<queue>)
        n157 = Unbundle By Name(w466) -> ("Configuration"=w465:T34)
        n158 = call "Enqueue Message (Single).vi"("error in (no error)"=w473, "Message"="Notify Status", "Message Queue"=w484) -> ("error out"=w474:errorcluster)  [unwired: 1 in, 7 out]
        n159 = Merge Errors(w475, w474) -> (w482:errorcluster)
      }
      frame "Add Instrument Sequence Step" {
        n160 = Unbundle By Name(w502) -> ("Instrument Sequence.Instrument Data"=w501:refnum<notifier>)
        n161 = Unbundle By Name(w505) -> ("Instrument Sequence"=w507:refnum<queue>)
        n162 = Cancel Notification(0:w501, 3:w504) -> (8:w491:refnum<notifier>, 11:w492:errorcluster)  [unwired: 1 out]
        n163 = Wait on Notification(notifier=w491, error in (no error)=w492) -> (notification=w500:variant, error out=w503:errorcluster)  [unwired: 4 out]
        n164 = call "Enqueue Message (Single).vi"("error in (no error)"=w492, "Message"="Add Step", "Message Queue"=w507) -> ("error out"=w489:errorcluster)  [unwired: 1 in, 7 out]
        n165 = Merge Errors(w489, w503) -> (w490:errorcluster)
        n166 = Variant To Data(error in=w490, type=T2 [] ("Instrument Steps 2"), Variant=w500) -> (data=w493:T2, error out=w488:errorcluster)
        n167 = Unbundle By Name(w494) -> ("Instrument Steps"=w498:refnum<vi>)
        n168 = Not A Number/Path/Refnum?(number/path/refnum=w498) -> (NaN/Path/Refnum?=w497:bool)
        n169 = case shown="False" w497 {
          tunnel: w498 -> [w515 _]
          tunnel: w493 -> [w514 _]
          tunnel: w488 -> [w513 w516]
          tunnel: [w512 w516] -> w487
          frame False {
            n170 = property class="Arr (strict)"(reference=w515, error in=w513, "Value"=w514) -> (error out=w512:errorcluster)  [unwired: 1 out]
          }
          frame True {
          }
        }
      }
      frame "Delete Instrument Sequence Step" {
        n171 = Unbundle By Name(w532) -> ("Instrument Sequence.Instrument Data"=w531:refnum<notifier>)
        n172 = Unbundle By Name(w535) -> ("Instrument Sequence"=w537:refnum<queue>)
        n173 = Cancel Notification(0:w531, 3:w534) -> (8:w521:refnum<notifier>, 11:w522:errorcluster)  [unwired: 1 out]
        n174 = Wait on Notification(notifier=w521, error in (no error)=w522) -> (notification=w530:variant, error out=w533:errorcluster)  [unwired: 4 out]
        n175 = call "Enqueue Message (Single).vi"("error in (no error)"=w522, "Message"="Remove Step", "Message Queue"=w537) -> ("error out"=w519:errorcluster)  [unwired: 1 in, 7 out]
        n176 = Merge Errors(w519, w533) -> (w520:errorcluster)
        n177 = Variant To Data(error in=w520, type=T2 [] ("Instrument Steps 2"), Variant=w530) -> (data=w523:T2, error out=w518:errorcluster)
        n178 = Unbundle By Name(w524) -> ("Instrument Steps"=w528:refnum<vi>)
        n179 = Not A Number/Path/Refnum?(number/path/refnum=w528) -> (NaN/Path/Refnum?=w527:bool)
        n180 = case shown="False" w527 {
          tunnel: w528 -> [w545 _]
          tunnel: w523 -> [w544 _]
          tunnel: w518 -> [w543 w546]
          tunnel: [w542 w546] -> w517
          frame False {
            n181 = property class="Arr (strict)"(reference=w545, error in=w543, "Value"=w544) -> (error out=w542:errorcluster)  [unwired: 1 out]
          }
          frame True {
          }
        }
      }
      frame "Clear Instrument Sequence" {
        n182 = Unbundle By Name(w562) -> ("Instrument Sequence.Instrument Data"=w561:refnum<notifier>)
        n183 = Cancel Notification(0:w561, 3:w564) -> (8:w551:refnum<notifier>, 11:w552:errorcluster)  [unwired: 1 out]
        n184 = Unbundle By Name(w565) -> ("Instrument Sequence"=w567:refnum<queue>)
        n185 = Wait on Notification(notifier=w551, error in (no error)=w552) -> (notification=w560:variant, error out=w563:errorcluster)  [unwired: 4 out]
        n186 = call "Enqueue Message (Single).vi"("error in (no error)"=w552, "Message"="Clear Sequence", "Message Queue"=w567) -> ("error out"=w549:errorcluster)  [unwired: 1 in, 7 out]
        n187 = Merge Errors(w549, w563) -> (w550:errorcluster)
        n188 = Variant To Data(error in=w550, type=T2 [] ("Instrument Steps 2"), Variant=w560) -> (data=w553:T2, error out=w548:errorcluster)
        n189 = Unbundle By Name(w554) -> ("Instrument Steps"=w558:refnum<vi>)
        n190 = Not A Number/Path/Refnum?(number/path/refnum=w558) -> (NaN/Path/Refnum?=w557:bool)
        n191 = case shown="False" w557 {
          tunnel: w558 -> [w575 _]
          tunnel: w553 -> [w574 _]
          tunnel: w548 -> [w573 w576]
          tunnel: [w572 w576] -> w547
          frame False {
            n192 = property class="Arr (strict)"(reference=w575, error in=w573, "Value"=w574) -> (error out=w572:errorcluster)  [unwired: 1 out]
          }
          frame True {
          }
        }
      }
      frame "Load Instrument Sequence" {
        n193 = Unbundle By Name(w592) -> ("Instrument Sequence.Instrument Data"=w591:refnum<notifier>)
        n194 = Cancel Notification(0:w591, 3:w594) -> (8:w581:refnum<notifier>, 11:w582:errorcluster)  [unwired: 1 out]
        n195 = Unbundle By Name(w595) -> ("Instrument Sequence"=w597:refnum<queue>)
        n196 = Wait on Notification(notifier=w581, error in (no error)=w582) -> (notification=w590:variant, error out=w593:errorcluster)  [unwired: 4 out]
        n197 = call "Enqueue Message (Single).vi"("error in (no error)"=w582, "Message"="Load Sequence", "Message Queue"=w597) -> ("error out"=w579:errorcluster)  [unwired: 1 in, 7 out]
        n198 = Merge Errors(w579, w593) -> (w580:errorcluster)
        n199 = Variant To Data(error in=w580, type=T2 [] ("Instrument Steps 2"), Variant=w590) -> (data=w583:T2, error out=w578:errorcluster)
        n200 = Unbundle By Name(w584) -> ("Instrument Steps"=w588:refnum<vi>)
        n201 = Not A Number/Path/Refnum?(number/path/refnum=w588) -> (NaN/Path/Refnum?=w587:bool)
        n202 = case shown="False" w587 {
          tunnel: w588 -> [w605 _]
          tunnel: w583 -> [w604 _]
          tunnel: w578 -> [w603 w606]
          tunnel: [w602 w606] -> w577
          frame False {
            n203 = property class="Arr (strict)"(reference=w605, error in=w603, "Value"=w604) -> (error out=w602:errorcluster)  [unwired: 1 out]
          }
          frame True {
          }
        }
      }
      frame "Reset Instrument Sequence" {
        n204 = Unbundle By Name(w619) -> ("Instrument Sequence.Instrument Data"=w617:refnum<notifier>)
        n205 = Cancel Notification(0:w617, 3:w622) -> (11:w618:errorcluster)  [unwired: 2 out]
        n206 = Unbundle By Name(w623) -> ("Instrument Sequence"=w625:refnum<queue>)
        n207 = call "Enqueue Message (Single).vi"("error in (no error)"=w618, "Message"="Reset Sequence", "Message Queue"=w625) -> ("error out"=w621:errorcluster)  [unwired: 1 in, 7 out]
        n208 = Wait on Notification(notifier=w617, error in (no error)=w621) -> (notification=w616:variant, error out=w620:errorcluster)  [unwired: 4 out]
        n209 = Variant To Data(error in=w620, type=T2 [] ("Instrument Steps 2"), Variant=w616) -> (data=w607:T2, error out=w612:errorcluster)
        n210 = Unbundle By Name(w610) -> ("Instrument Steps"=w614:refnum<vi>)
        n211 = Not A Number/Path/Refnum?(number/path/refnum=w614) -> (NaN/Path/Refnum?=w613:bool)
        n212 = case shown="False" w613 {
          tunnel: w614 -> [w633 _]
          tunnel: w607 -> [w632 _]
          tunnel: w612 -> [w631 w634]
          tunnel: [w630 w634] -> w611
          frame False {
            n213 = property class="Arr (strict)"(reference=w633, error in=w631, "Value"=w632) -> (error out=w630:errorcluster)  [unwired: 1 out]
          }
          frame True {
          }
        }
      }
      frame "Save Instrument Sequence" {
        n214 = Unbundle By Name(w646) -> ("Instrument Sequence.Status"=w645:refnum<notifier>)
        n215 = Cancel Notification(0:w645, 3:w647) -> (8:w640:refnum<notifier>, 11:w638:errorcluster)  [unwired: 1 out]
        n216 = Unbundle By Name(w648) -> ("Instrument Sequence"=w650:refnum<queue>)
        n217 = call "Enqueue Message (Single).vi"("error in (no error)"=w638, "Message"="Save Sequence", "Message Queue"=w650) -> ("error out"=w635:errorcluster)  [unwired: 1 in, 7 out]
        n218 = call "Wait for event.vi"("error in (no error)"=w638, "String"="Instrument Sequence Saved" ("Message"), "Notifier in"=w640) -> ("error out"=w637:errorcluster)  [unwired: 7 in, 1 out]
        n219 = Merge Errors(w635, w637) -> (w636:errorcluster)
      }
      frame "Pause" {
        n220 = Unbundle By Name(w659) -> ("Pause-Resume"=w658:refnum<vi>)
        n221 = call "Pause.vi"("error in (no error)"=w660, "Pause-Resume"=w658) -> ("error out"=w661:errorcluster)  [unwired: 9 out]
      }
      frame "Stop" {
        n222 = Unbundle By Name(w670) -> ("Strain Measurement"=w672:refnum<queue>)
        n223 = Flush Queue(queue=w672, error in (no error)=w671) -> (error out=w668:errorcluster)  [unwired: 2 out]
      }
    }
  }
  "error out" <- w5
  "Sequence Progress" <- w4
  "Instrument Steps" <- w3
